vi "scope.vi"() -> ()   [LabVIEW 2017]
uses:
  <vilib>/FPGAPlugInAG/myRIO-1900/niLvFpga_Open_myRIO-1900.vi
  <vilib>/rvi/interface/common/dynamic/niFpgaDynamicAddResources.vi
  <vilib>/rvi/interface/common/niFpgaWaitOnOcc.vi
  <vilib>/Utility/error.llb/Error Cluster From Error Code.vi
  <vilib>/express/express shared/transition.llb/Dynamic To Waveform Array.vi
  <vilib>/express/express signal manip/GetorSetDDTAttributes/Set DDT Attributes/SetT0.vi
  <vilib>/express/express shared/transition.llb/Waveform Array To Dynamic.vi
  <vilib>/rvi/errors/niLvFpgaAdjustHostInterfaceError.vi
  <vilib>/FPGAPlugInAG/Dynamic/niLvFpga_Close_Dynamic.vi
  <vilib>/rvi/interface/nirviOpenFPGA/nirviOpenFPGA.xnode
  FPGA Bitfiles/testznakowarki_FPGATarget_readtescior_VLrWmtzxVOU.lvbitx
  read_and_write.vi
  <vilib>/rvi/interface/nirviMethod/nirviMethod.xnode
  <vilib>/express/express signal manip/GetorSetDDTAttributes/Set DDT Attributes/Set DDT Properties.xnode
  <vilib>/rvi/interface/nirviReadWriteControl/nirviReadWriteControl.xnode
  <vilib>/rvi/interface/nirviCloseFPGA/nirviCloseFPGA.xnode
  <vilib>/rvi/errors/niLvFpgaMergeErrorWithErrorCode.vi
  <vilib>/rvi/interface/Simulation/niFpgaSimulationCallBeginRW.vi
  NiFpgaLv.dll
  <vilib>/FPGAPlugInAG/Dynamic/niLvFpga_ConfigureFifo_Dynamic.vi
  <vilib>/FPGAPlugInAG/Dynamic/niLvFpga_ReadFifo_Dynamic.vi
panel:
  out "Numeric":i32
  out "trigger count queue":i16
  out "inqueue":i32[][](array[numeric])
  in  "stop":bool
  in  "Tab Control":enum32{"now", "data", "settings"}(tab)=enum."settings"
  out "?":string="error now"
  out "error x":bool=TRUE
  out "error y":bool=TRUE
  out "?":string="error now"
  out "max/min x":bool=TRUE
  out "max/min y":bool=TRUE
  out "deviation error x":bool=TRUE
  out "deviation error y":bool=TRUE
  out "data graph":cluster{"time":i32[], "data y":i16[]}[](graph)
  out "template graph":cluster{"time":i32[], "data y":i16[]}[](graph)
  out "size now":i32=2439
  out "max x now":i16=-144
  out "min x now":i16=-150
  out "max y now":i16=116
  out "min y now":i16=-99
  out "template size":i32=10156
  out "template min x":i16=-154
  out "template max x":i16=152
  out "template min y":i16=-135
  out "template max y":i16=139
  out "deviation x":dbl=5341.338663386656
  out "deviation y":dbl=10700.440754407726
  out "template":bool=TRUE
  out "trigger":bool
  out "trigger count":i16=7
  in  "data x":i16[](array[numeric])=[-148, -149, -148, -148, -148, -149, -148, -149, -148, -149, -146, -148, -148, -150, -148, -148, -149, -148, -147, -148, -149, -147, -149, -147, -148, -148, -149, -149, -148, -148, -149, -148, -149, -149, -148, -148, -148, -149, -148, -148, -149, -149, -148, -148, -149, -148, -147, -148, -148, -148, -149, -148, -148, -148, -148, -147, -149, -148, -148, -148, -149, -148, -149, -148, -148, -148, -148, -149, -148, -148, -147, -148, -148, -149, -148, -149, -148, -148, -148, -148, -148, -148, -149, -148, -148, -149, -149, -148, -148, -149, -149, -148, -149, -146, -148, -148, -149, -148, -148, -148, -148, -148, -148, -149, -148, -149, -148, -148, -148, -148, -148, -149, -148, -149, -148, -149, -148, -148, -148, -149, -149, -149, -148, -148, -149, -148, -149, -148, -149, -149, -146, -149, -148, -149, -149, -148, -148, -149, -149, -148, -146, -148, -150, -148, -148, -148, -147, -149, -148, -148, -148, -149, -147, -148, -148, -148, -148, -149, -149, -148, -147, -148, -148, -147, -149, -149, -147, -149, -147, -148, -149, -149, -148, -149, -148, -148, -148, -149, -149, -148, -149, -147, -147, -148, -149, -149, -147, -149, -148, -148, -149, -150, -148, -148, -149, -148, -149, -149, -149, -146, -148, -148, -148, -148, -149, -148, -148, -147, -148, -148, -149, -149, -148, -148, -149, -147, -148, -149, -147, -148, -149, -149, -149, -149, -148, -148, -149, -149, -148, -148, -149, -147, -149, -148, -148, -148, -148, -149, -148, -148, -148, -148, -149, -148, -148, -149, -148, -149, -149, -148, -148, -147, -149, -149, -148, -149, -149, -148, -148, -147, -149, -148, -148, -149, -148, -149, -148, -148, -148, -149, -149, -149, -144, -149, -148, -149, -149, -148, -148, -148, -148, -149, -147, -149, -148, -149, -148, -146, -149, -148, -148, -148, -148, -149, -149, -148, -149, -148, -149, -148, -148, -148, -148, -149, -149, -148, -149, -148, -149, -147, -148, -148, -148, -149, -149, -147, -148, -148, -149, -147, -148, -148, -149, -148, -148, -147, -148, -148, -149, -147, -148, -149, -149, -149, -145, -149, -149, -148, -148, -148, -149, -148, -147, -149, -148, -149, -148, -148, -149, -146, -148, -149, -148, -149, -148, -149, -148, -148, -149, -149, -148, -149, -149, -149, -148, -148, -149, -148, -149, -147, -148, -148, -148, -145, -149, -148, -148, -148, -149, -148, -149, -149, -148, -147, -149, -149, -147, -149, -149, -147, -148, -149, -149, -148, -148, -149, -146, -148, -148, -148, -149, -148, -148, -148, -149, -148, -149, -149, -148, -148, -147, -149, -148, -148, -148, -148, -148, -148, -148, -149, -146, -149, -147, -149, -149, -149, -148, -148, -149, -148, -149, -148, -148, -148, -147, -149, -148, -148, -149, -149, -149, -147, -148, -148, -149, -146, -148, -149, -147, -148, -149, -146, -148, -148, -148, -148, -148, -149, -148, -148, -148, -147, -148, -149, -148, -147, -148, -148, -149, -148, -149, -149, -148, -148, -148, -148, -148, -148, -148, -149, -149, -148, -149, -148, -147, -148, -149, -148, -149, -149, -149, -148, -149, -148, -148, -148, -148, -148, -145, -149, -149, -148, -148, -148, -148, -149, -149, -148, -147, -149, -149, -148, -148, -149, -148, -149, -148, -149, -149, -148, -149, -148, -148, -150, -146, -149, -148, -149, -149, -149, -149, -146, -148, -149, -148, -149, -149, -148, -148, -149, -148, -149, -148, -148, -149, -149, -147, -148, -148, -148, -148, -148, -149, -148, -148, -148, -149, -148, -150, -148, -148, -148, -147, -148, -149, -148, -148, -148, -148, -149, -148, -149, -148, -148, -149, -149, -148, -148, -148, -149, -148, -149, -149, -148, -149, -149, -148, -148, -147, -150, -148, -149, -148, -148, -148, -149, -148, -148, -148, -146, -148, -149, -148, -148, -148, -149, -148, -148, -148, -147, -148, -149, -148, -148, -148, -148, -148, -149, -147, -148, -148, -149, -149, -148, -148, -148, -147, -149, -148, -149, -148, -148, -149, -148, -149, -148, -149, -149, -149, -148, -147, -148, -148, -148, -149, -148, -148, -149, -148, -149, -148, -149, -148, -148, -148, -148, -147, -148, -148, -149, -148, -150, -148, -148, -149, -149, -146, -149, -149, -148, -149, -148, -148, -148, -147, -148, -148, -148, -148, -148, -148, -149, -148, -149, -148, -148, -149, -147, -148, -149, -148, -148, -148, -149, -149, -148, -149, -148, -149, -148, -146, -148, -148, -148, -149, -147, -149, -150, -148, -149, -149, -148, -149, -148, -149, -149, -148, -149, -148, -149, -149, -146, -149, -148, -148, -148, -149, -149, -147, -149, -149, -148, -149, -149, -148, -149, -149, -150, -148, -148, -149, -148, -148, -149, -148, -149, -149, -149, -149, -147, -148, -147, -148, -148, -148, -149, -148, -149, -148, -149, -148, -148, -149, -148, -148, -149, -148, -150, -148, -149, -148, -149, -148, -148, -149, -148, -148, -149, -146, -148, -148, -148, -148, -149, -149, -149, -149, -149, -147, -148, -149, -149, -149, -148, -149, -148, -149, -149, -149, -148, -148, -149, -149, -148, -149, -148, -148, -149, -149, -148, -147, -148, -149, -147, -149, -148, -148, -149, -147, -148, -149, -148, -148, -148, -149, -148, -148, -148, -149, -147, -149, -148, -149, -148, -148, -146, -148, -149, -148, -148, -148, -149, -148, -148, -149, -149, -147, -149, -150, -147, -148, -149, -148, -149, -149, -149, -146, -149, -148, -148, -148, -149, -149, -147, -148, -149, -147, -149, -148, -148, -150, -149, -148, -149, -148, -149, -149, -149, -147, -149, -148, -149, -147, -149, -149, -149, -148, -148, -148, -147, -148, -148, -147, -149, -149, -148, -148, -149, -148, -148, -149, -147, -149, -146, -148, -148, -148, -150, -148, -149, -149, -147, -149, -148, -148, -148, -150, -148, -148, -149, -149, -148, -149, -148, -148, -147, -149, -148, -148, -148, -149, -149, -148, -149, -148, -147, -148, -148, -148, -148, -149, -148, -149, -149, -148, -148, -149, -148, -147, -150, -147, -149, -148, -149, -148, -149, -149, -149, -149, -149, -148, -149, -148, -150, -148, -149, -148, -146, -149, -149, -148, -149, -149, -149, -149, -148, -150, -148, -148, -148, -148, -148, -149, -148, -149, -149, -148, -149, -148, -148, -148, -147, -149, -148, -149, -148, -148, -149, -149, -148, -148, -148, -148, -148, -148, -148, -148, -148, -149, -148, -149, -148, -148, -148, -147, -148, -149, -149, -148, -147, -149, -149, -148, -148, -146, -148, -148, -149, -149, -148, -149, -148, -148, -149, -148, -149, -147, -149, -146, -148, -148, -148, -147, -149, -149, -147, -149, -149, -148, -148, -148, -149, -147, -148, -148, -148, -148, -148, -149, -148, -148, -148, -149, -149, -149, -149, -149, -148, -148, -148, -149, -148, -149, -149, -148, -148, -148, -149, -148, -148, -148, -148, -149, -149, -148, -147, -148, -148, -148, -149, -147, -148, -148, -147, -147, -148, -148, -149, -147, -149, -145, -148, -148, -149, -148, -149, -148, -148, -148, -149, -148, -148, -148, -149, -148, -147, -148, -148, -149, -148, -149, -148, -148, -148, -149, -146, -148, -148, -149, -148, -148, -149, -149, -147, -149, -148, -149, -149, -148, -148, -148, -149, -148, -148, -149, -149, -148, -149, -148, -149, -148, -149, -149, -147, -148, -149, -147, -149, -149, -148, -148, -147, -147, -148, -149, -147, -147, -149, -149, -148, -149, -149, -148, -148, -148, -149, -148, -149, -147, -148, -146, -149, -148, -148, -148, -149, -148, -149, -148, -148, -149, -148, -148, -149, -148, -148, -149, -148, -148, -148, -149, -148, -148, -147, -148, -148, -150, -149, -148, -148, -149, -148, -149, -148, -148, -148, -146, -148, -147, -148, -149, -148, -150, -148, -149, -147, -150, -148, -148, -149, -149, -148, -149, -148, -149, -146, -148, -148, -148, -148, -149, -149, -146, -148, -149, -148, -149, -148, -147, -149, -149, -148, -148, -148, -148, -148, -148, -148, -148, -148, -149, -149, -148, -146, -148, -149, -148, -148, -148, -149, -149, -147, -149, -148, -147, -149, -148, -148, -148, -148, -148, -150, -145, -148, -148, -148, -148, -149, -149, -148, -147, -148, -148, -148, -148, -148, -149, -148, -148, -148, -149, -148, -149, -148, -147, -149, -148, -148, -149, -148, -148, -149, -149, -148, -148, -147, -149, -148, -149, -148, -148, -148, -149, -148, -148, -148, -148, -147, -149, -148, -148, -148, -149, -148, -148, -148, -148, -148, -148, -148, -148, -147, -148, -148, -149, -149, -148, -149, -149, -148, -149, -147, -148, -149, -147, -149, -148, -148, -149, -148, -149, -149, -148, -149, -147, -148, -148, -149, -149, -147, -147, -148, -147, -149, -148, -147, -150, -149, -146, -148, -148, -149, -148, -149, -148, -148, -148, -148, -148, -149, -149, -149, -148, -148, -148, -145, -148, -149, -149, -148, -149, -149, -148, -149, -149, -147, -148, -149, -147, -149, -148, -148, -148, -149, -149, -148, -150, -145, -149, -148, -147, -148, -149, -149, -147, -148, -149, -148, -148, -148, -149, -147, -148, -148, -148, -147, -148, -149, -148, -147, -149, -148, -146, -148, -148, -148, -149, -149, -148, -148, -149, -147, -147, -149, -148, -147, -149, -148, -149, -148, -149, -148, -149, -149, -149, -148, -148, -148, -148, -148, -150, -147, -149, -148, -149, -148, -148, -149, -148, -146, -148, -148, -149, -146, -148, -148, -149, -149, -148, -149, -148, -148, -148, -148, -148, -149, -148, -148, -149, -148, -148, -149, -149, -149, -148, -148, -148, -148, -148, -149, -148, -148, -148, -149, -148, -148, -149, -149, -148, -148, -148, -148, -148, -148, -148, -148, -149, -148, -149, -149, -147, -148, -148, -147, -149, -148, -148, -147, -149, -149, -148, -148, -149, -146, -148, -148, -147, -148, -148, -149, -148, -149, -149, -146, -148, -148, -149, -149, -149, -145, -148, -148, -149, -148, -148, -149, -148, -148, -148, -149, -148, -148, -149, -149, -148, -149, -148, -148, -148, -148, -149, -148, -148, -148, -146, -149, -148, -148, -149, -147, -148, -148, -148, -149, -148, -149, -149, -148, -149, -149, -146, -148, -149, -149, -148, -150, -148, -147, -149, -148, -149, -148, -149, -149, -147, -148, -149, -148, -148, -148, -149, -146, -149, -149, -149, -148, -148, -148, -149, -149, -148, -147, -149, -148, -148, -148, -148, -148, -148, -149, -149, -148, -148, -148, -146, -149, -147, -149, -148, -149, -148, -149, -149, -148, -148, -149, -147, -149, -148, -149, -149, -149, -148, -148, -148, -148, -148, -149, -146, -149, -149, -149, -148, -149, -148, -149, -148, -149, -149, -147, -149, -150, -149, -148, -149, -147, -147, -148, -149, -148, -148, -150, -147, -148, -149, -148, -149, -148, -149, -148, -148, -148, -148, -148, -148, -149, -148, -149, -148, -149, -149, -147, -148, -148, -149, -148, -149, -149, -148, -147, -149, -148, -146, -148, -148, -149, -148, -149, -148, -149, -148, -149, -145, -148, -148, -149, -148, -149, -149, -148, -148, -148, -147, -148, -148, -148, -149, -148, -149, -147, -149, -148, -148, -149, -148, -148, -148, -147, -149, -148, -149, -148, -148, -149, -148, -148, -148, -148, -148, -148, -149, -149, -149, -147, -149, -150, -149, -148, -148, -147, -149, -148, -150, -148, -149, -148, -148, -147, -148, -148, -148, -149, -148, -149, -149, -149, -147, -148, -149, -148, -148, -149, -149, -147, -147, -149, -148, -148, -148, -149, -146, -148, -148, -149, -148, -148, -148, -149, -148, -147, -148, -148, -148, -149, -148, -148, -149, -148, -148, -150, -148, -148, -149, -147, -148, -149, -149, -147, -149, -148, -148, -149, -149, -149, -148, -149, -149, -148, -148, -149, -149, -147, -149, -148, -149, -149, -149, -147, -148, -149, -149, -147, -149, -147, -148, -148, -149, -147, -149, -148, -150, -148, -149, -148, -148, -149, -148, -149, -148, -149, -148, -148, -149, -148, -147, -148, -148, -148, -148, -149, -148, -148, -147, -149, -148, -149, -148, -148, -149, -148, -149, -148, -149, -148, -148, -149, -148, -149, -149, -148, -148, -146, -148, -149, -149, -148, -148, -149, -149, -148, -147, -148, -149, -148, -149, -149, -148, -147, -149, -149, -148, -147, -148, -148, -148, -147, -148, -147, -148, -148, -148, -148, -148, -147, -149, -149, -145, -149, -149, -148, -148, -148, -149, -148, -149, -149, -148, -149, -148, -148, -148, -149, -148, -149, -147, -149, -148, -149, -147, -147, -149, -149, -148, -148, -148, -149, -148, -148, -149, -149, -147, -149, -148, -148, -148, -149, -147, -148, -148, -148, -148, -149, -150, -145, -149, -149, -148, -148, -150, -148, -148, -149, -149, -148, -149, -148, -149, -148, -150, -149, -148, -148, -149, -148, -149, -148, -149, -147, -149, -148, -148, -149, -148, -148, -149, -148, -148, -148, -148, -147, -149, -148, -149, -148, -149, -148, -148, -148, -148, -148, -148, -149, -149, -148, -149, -148, -146, -148, -150, -149, -149, -148, -149, -149, -148, -149, -149, -148, -150, -147, -148, -149, -149, -148, -148, -149, -149, -148, -149, -146, -147, -149, -148, -148, -147, -149, -149, -147, -149, -148, -149, -149, -148, -147, -149, -148, -148, -148, -149, -149, -148, -148, -148, -147, -148, -148, -149, -148, -149, -148, -147, -148, -149, -148, -149, -149, -147, -149, -149, -148, -149, -149, -149, -148, -148, -148, -147, -149, -149, -149, -148, -147, -148, -148, -148, -149, -147, -149, -147, -148, -149, -148, -148, -149, -148, -149, -146, -149, -148, -148, -149, -148, -148, -148, -148, -148, -148, -146, -148, -148, -148, -149, -148, -149, -148, -148, -148, -148, -148, -148, -148, -149, -148, -149, -148, -148, -148, -149, -150, -147, -149, -149, -148, -148, -150, -145, -148, -149, -149, -148, -149, -149, -148, -147, -149, -148, -148, -149, -148, -148, -148, -148, -148, -148, -148, -149, -148, -149, -148, -148, -148, -148, -149, -147, -148, -148, -148, -147, -149, -148, -148, -148, -149, -148, -148, -149, -148, -148, -149, -148, -148, -149, -148, -148, -148, -149, -148, -148, -148, -147, -149, -149, -148, -148, -149, -146, -148, -149, -147, -149, -148, -149, -148, -148, -149, -149, -148, -148, -147, -148, -148, -149, -148, -148, -148, -149, -149, -148, -147, -148, -150, -148, -148, -147, -149, -148, -149, -148, -149, -148, -149, -149, -148, -149, -149, -147, -148, -148, -148, -148, -149, -148, -148, -148, -149, -147, -148, -149, -149, -149, -148, -148, -148, -148, -148, -146, -148, -149, -148, -149, -147, -148, -148, -148, -149, -147, -149, -148, -148, -149, -147, -148, -148, -148, -149, -148, -148, -149, -146, -149, -149, -148, -148, -148, -150, -146, -149, -149, -148, -148, -148, -148, -148, -149, -148, -150, -146, -149, -148, -149, -148, -148, -148, -149, -147, -149, -148, -149, -148, -146, -148, -149, -148, -149, -149, -148, -148, -149, -148, -149, -148, -149, -149, -149, -148, -145, -149, -149, -149, -149, -149, -149, -147, -148, -148, -148, -149, -149, -149, -149, -148, -148, -148, -148, -148, -149, -148, -149, -148, -149, -148, -148, -148, -149, -148, -148, -147, -148, -148, -148, -148, -148, -150, -149, -148, -149, -148, -148, -149, -148, -148, -148, -148, -148, -148, -148, -149, -148, -148, -149, -147, -148, -149, -149, -148, -149, -149, -146, -148, -148, -149, -148, -148, -149, -148, -148, -149, -145, -150]
  in  "data y":i16[](array[numeric])=[-99, -98, -98, -98, -98, -98, -97, -98, -97, -97, -97, -97, -96, -98, -97, -97, -96, -97, -96, -97, -97, -96, -95, -97, -96, -95, -96, -97, -96, -96, -96, -95, -95, -95, -95, -93, -95, -96, -95, -95, -96, -95, -94, -95, -95, -94, -94, -94, -94, -94, -94, -94, -94, -93, -93, -91, -94, -93, -92, -94, -94, -93, -93, -91, -93, -92, -93, -91, -92, -92, -92, -92, -92, -92, -92, -91, -91, -91, -91, -91, -93, -91, -91, -91, -91, -92, -91, -90, -91, -88, -91, -91, -90, -90, -89, -91, -89, -89, -89, -90, -89, -89, -90, -88, -89, -88, -89, -88, -89, -89, -86, -89, -89, -88, -89, -89, -87, -88, -88, -87, -87, -88, -89, -87, -87, -87, -85, -87, -87, -88, -87, -87, -87, -86, -86, -87, -84, -87, -87, -86, -86, -87, -86, -85, -85, -87, -85, -85, -85, -85, -85, -85, -84, -85, -85, -85, -85, -83, -85, -84, -83, -84, -84, -85, -84, -84, -83, -82, -84, -83, -83, -83, -81, -84, -83, -82, -82, -83, -83, -83, -83, -83, -82, -82, -82, -82, -83, -82, -82, -81, -82, -82, -81, -82, -81, -81, -81, -81, -81, -81, -81, -82, -81, -82, -81, -79, -80, -80, -80, -80, -80, -80, -79, -80, -77, -79, -80, -80, -79, -80, -79, -79, -79, -80, -78, -78, -79, -77, -78, -77, -79, -78, -79, -80, -77, -77, -78, -77, -77, -78, -77, -76, -78, -78, -78, -74, -78, -76, -76, -77, -77, -76, -75, -76, -76, -76, -76, -76, -76, -75, -76, -76, -76, -76, -76, -75, -75, -74, -75, -74, -75, -76, -75, -75, -73, -75, -74, -74, -74, -74, -73, -74, -74, -74, -74, -73, -74, -73, -73, -73, -72, -74, -70, -74, -72, -72, -73, -73, -73, -71, -71, -72, -72, -72, -72, -71, -72, -71, -71, -72, -71, -71, -71, -71, -71, -70, -71, -71, -71, -70, -71, -70, -71, -70, -70, -70, -70, -69, -70, -69, -69, -70, -69, -69, -69, -69, -69, -69, -69, -69, -69, -69, -69, -68, -68, -69, -68, -68, -68, -68, -67, -68, -68, -68, -67, -68, -66, -67, -67, -67, -66, -67, -65, -66, -67, -67, -66, -66, -67, -66, -65, -66, -64, -65, -66, -66, -66, -66, -66, -65, -65, -64, -65, -64, -65, -64, -64, -65, -65, -64, -64, -64, -64, -64, -64, -64, -63, -64, -63, -64, -64, -64, -62, -64, -63, -63, -63, -64, -62, -63, -62, -63, -62, -63, -62, -62, -60, -62, -62, -62, -62, -62, -60, -62, -62, -61, -62, -58, -60, -61, -61, -61, -61, -62, -59, -59, -61, -60, -61, -60, -60, -60, -57, -59, -60, -59, -60, -59, -60, -59, -59, -58, -59, -59, -59, -57, -59, -59, -58, -57, -58, -58, -58, -56, -58, -57, -58, -57, -58, -57, -58, -56, -57, -57, -56, -56, -57, -57, -57, -57, -57, -56, -55, -56, -56, -56, -57, -56, -57, -53, -56, -55, -56, -55, -53, -55, -55, -55, -54, -54, -55, -54, -54, -55, -54, -54, -54, -54, -53, -54, -54, -54, -53, -54, -53, -54, -53, -54, -53, -53, -53, -53, -52, -53, -52, -53, -53, -52, -52, -53, -52, -52, -52, -52, -51, -53, -52, -52, -52, -52, -50, -51, -51, -52, -52, -51, -51, -50, -50, -51, -50, -49, -50, -49, -50, -49, -49, -50, -50, -50, -50, -48, -49, -48, -49, -49, -49, -49, -48, -49, -47, -49, -49, -47, -48, -48, -47, -48, -48, -48, -48, -48, -48, -47, -47, -48, -47, -47, -47, -47, -46, -48, -47, -47, -46, -47, -46, -47, -47, -47, -45, -47, -45, -46, -45, -45, -45, -44, -45, -43, -44, -45, -44, -43, -45, -45, -44, -43, -44, -44, -44, -45, -45, -45, -42, -44, -44, -44, -44, -43, -44, -44, -42, -42, -44, -43, -43, -43, -43, -42, -43, -42, -42, -42, -42, -43, -42, -42, -42, -41, -42, -41, -38, -41, -41, -40, -41, -41, -41, -40, -41, -41, -40, -41, -38, -40, -40, -40, -41, -40, -41, -38, -39, -40, -39, -39, -40, -40, -39, -38, -39, -40, -38, -38, -39, -38, -38, -39, -38, -37, -38, -39, -38, -38, -38, -37, -37, -38, -36, -38, -37, -38, -36, -38, -37, -37, -36, -37, -36, -37, -37, -36, -36, -36, -35, -36, -37, -36, -36, -35, -35, -36, -36, -35, -35, -35, -36, -35, -35, -34, -33, -34, -35, -35, -34, -34, -34, -33, -34, -34, -32, -34, -34, -33, -33, -33, -34, -33, -33, -33, -33, -33, -33, -31, -33, -33, -32, -32, -32, -30, -32, -31, -32, -32, -31, -32, -32, -32, -31, -31, -31, -31, -31, -30, -31, -31, -31, -30, -30, -31, -31, -30, -29, -30, -30, -30, -29, -29, -29, -30, -27, -29, -29, -29, -29, -29, -28, -28, -29, -28, -26, -29, -29, -29, -28, -30, -26, -28, -27, -27, -27, -27, -28, -28, -26, -27, -28, -27, -27, -26, -28, -24, -26, -27, -26, -27, -26, -26, -26, -25, -26, -25, -26, -26, -26, -25, -25, -25, -25, -24, -26, -23, -25, -25, -25, -24, -24, -24, -25, -23, -25, -25, -24, -24, -24, -24, -23, -23, -24, -23, -23, -21, -23, -24, -22, -23, -22, -23, -20, -22, -22, -24, -21, -22, -23, -22, -22, -22, -19, -22, -21, -22, -21, -21, -22, -20, -21, -22, -20, -21, -20, -19, -19, -21, -21, -20, -20, -21, -20, -20, -20, -19, -20, -20, -19, -20, -19, -20, -18, -19, -20, -18, -18, -19, -19, -18, -19, -19, -18, -16, -19, -18, -18, -18, -18, -17, -17, -17, -18, -18, -17, -17, -14, -18, -17, -16, -16, -16, -17, -16, -16, -17, -14, -17, -15, -16, -16, -15, -16, -14, -15, -15, -16, -16, -15, -16, -15, -15, -14, -15, -14, -15, -15, -14, -14, -15, -14, -14, -13, -15, -13, -14, -13, -14, -13, -14, -13, -13, -13, -11, -12, -13, -13, -12, -13, -13, -12, -13, -12, -10, -11, -12, -12, -10, -12, -13, -8, -11, -11, -11, -11, -11, -12, -9, -10, -11, -10, -10, -11, -11, -8, -10, -9, -10, -10, -10, -11, -9, -9, -9, -8, -9, -9, -10, -9, -9, -9, -9, -9, -9, -9, -8, -9, -8, -9, -8, -8, -7, -8, -8, -6, -8, -9, -7, -8, -6, -7, -7, -6, -8, -6, -6, -7, -6, -7, -6, -7, -4, -5, -6, -7, -5, -6, -6, -6, -4, -6, -4, -5, -5, -4, -4, -6, -4, -5, -4, -5, -4, -5, -4, -1, -4, -5, -4, -3, -5, -3, -3, -3, -4, -3, -3, -3, -3, -2, -4, -1, -3, -2, -2, -2, -2, -2, -2, -2, -3, -2, -2, -2, -2, -1, 0, -2, -1, -2, -1, -1, -1, -1, -1, -1, 1, 0, -1, -1, 0, -1, -1, -1, 0, -1, 2, 0, 2, 0, 0, 1, 0, 2, 1, 1, 0, 1, 2, 1, 2, 3, 1, 2, 2, 1, 2, 2, 3, 2, 2, 3, 2, 5, 3, 2, 3, 3, 3, 3, 3, 4, 3, 4, 4, 3, 3, 4, 4, 4, 4, 4, 3, 7, 5, 4, 4, 5, 4, 4, 6, 6, 5, 6, 5, 5, 5, 6, 8, 6, 5, 6, 6, 6, 8, 6, 7, 7, 6, 7, 7, 6, 6, 7, 7, 7, 7, 8, 7, 8, 8, 7, 7, 8, 8, 7, 8, 8, 10, 8, 9, 8, 9, 9, 9, 8, 9, 9, 9, 9, 10, 8, 10, 9, 9, 10, 10, 10, 10, 10, 10, 12, 11, 11, 11, 10, 11, 10, 10, 11, 10, 11, 12, 11, 13, 11, 12, 11, 12, 12, 11, 12, 12, 12, 13, 12, 13, 13, 12, 12, 12, 13, 13, 13, 13, 16, 13, 13, 13, 14, 13, 14, 14, 15, 14, 15, 15, 15, 14, 15, 15, 14, 15, 15, 15, 17, 15, 15, 16, 15, 16, 17, 16, 15, 15, 16, 17, 15, 17, 15, 16, 20, 17, 17, 16, 17, 17, 17, 17, 17, 16, 17, 17, 20, 18, 17, 17, 17, 18, 17, 20, 19, 19, 17, 20, 18, 18, 18, 20, 19, 19, 19, 20, 19, 20, 19, 19, 20, 20, 19, 20, 19, 19, 20, 20, 20, 20, 20, 20, 20, 21, 20, 21, 21, 21, 22, 20, 22, 21, 20, 24, 21, 22, 23, 21, 22, 21, 23, 22, 22, 22, 23, 21, 23, 23, 23, 22, 24, 23, 26, 23, 25, 22, 23, 24, 23, 23, 23, 23, 24, 24, 25, 24, 25, 25, 25, 24, 25, 24, 25, 25, 25, 26, 25, 26, 26, 26, 26, 26, 26, 26, 26, 26, 25, 26, 26, 26, 26, 26, 26, 27, 26, 26, 29, 27, 27, 27, 28, 27, 27, 29, 27, 27, 28, 29, 28, 29, 28, 28, 30, 29, 28, 29, 29, 29, 28, 30, 29, 28, 29, 30, 29, 29, 30, 30, 29, 30, 30, 30, 30, 31, 30, 31, 31, 31, 30, 31, 30, 31, 31, 33, 31, 31, 31, 31, 32, 32, 32, 32, 32, 34, 32, 32, 31, 32, 33, 32, 33, 32, 34, 35, 33, 33, 33, 33, 36, 33, 34, 33, 34, 33, 32, 37, 34, 33, 35, 34, 35, 34, 35, 35, 33, 35, 35, 35, 35, 35, 35, 36, 35, 34, 35, 36, 35, 35, 35, 37, 36, 37, 36, 36, 38, 37, 37, 37, 37, 37, 37, 38, 37, 37, 36, 41, 37, 37, 38, 38, 37, 37, 40, 39, 38, 39, 38, 38, 38, 38, 41, 39, 38, 38, 39, 39, 39, 40, 40, 39, 39, 41, 41, 40, 41, 40, 39, 40, 41, 40, 40, 41, 42, 40, 43, 40, 41, 40, 42, 41, 41, 41, 42, 41, 41, 42, 42, 42, 42, 41, 42, 42, 42, 42, 42, 43, 42, 43, 43, 43, 43, 43, 44, 43, 44, 45, 43, 44, 44, 44, 44, 47, 44, 45, 44, 44, 44, 44, 44, 45, 44, 48, 45, 45, 45, 45, 45, 45, 45, 46, 45, 46, 45, 45, 47, 45, 46, 46, 46, 46, 47, 47, 48, 46, 47, 46, 47, 47, 48, 47, 48, 47, 50, 48, 48, 48, 47, 48, 48, 47, 48, 48, 49, 49, 49, 49, 48, 50, 48, 49, 49, 49, 49, 50, 49, 50, 49, 50, 51, 51, 50, 50, 50, 51, 49, 52, 50, 51, 50, 51, 51, 50, 53, 51, 51, 51, 52, 52, 52, 52, 51, 53, 51, 52, 52, 52, 52, 52, 52, 53, 53, 52, 54, 53, 53, 52, 53, 53, 53, 54, 54, 54, 54, 54, 53, 54, 54, 55, 54, 54, 55, 54, 57, 55, 54, 56, 54, 55, 55, 56, 55, 56, 55, 55, 55, 56, 56, 56, 55, 55, 57, 56, 57, 59, 57, 57, 57, 57, 57, 55, 56, 57, 56, 60, 57, 58, 58, 57, 57, 58, 58, 59, 58, 58, 57, 59, 58, 58, 58, 59, 59, 58, 59, 59, 59, 59, 59, 58, 60, 60, 59, 59, 60, 59, 60, 60, 60, 60, 61, 61, 63, 60, 61, 59, 61, 61, 61, 60, 62, 61, 64, 61, 62, 62, 61, 63, 62, 62, 63, 62, 65, 61, 63, 62, 62, 63, 63, 62, 63, 63, 63, 63, 63, 63, 63, 64, 63, 64, 64, 64, 63, 66, 64, 64, 64, 64, 64, 64, 65, 66, 64, 68, 65, 65, 66, 66, 65, 65, 66, 65, 64, 67, 66, 65, 66, 66, 65, 67, 67, 66, 67, 66, 67, 66, 67, 69, 67, 67, 68, 68, 68, 68, 68, 67, 68, 67, 68, 67, 68, 68, 68, 68, 69, 68, 69, 70, 69, 69, 70, 69, 68, 71, 69, 69, 70, 69, 69, 69, 71, 70, 70, 71, 70, 69, 70, 72, 71, 70, 71, 72, 71, 71, 73, 71, 72, 72, 71, 73, 71, 74, 72, 72, 73, 72, 72, 72, 72, 73, 71, 73, 72, 72, 74, 73, 73, 73, 73, 74, 74, 73, 74, 73, 75, 73, 74, 74, 73, 74, 75, 73, 75, 74, 75, 74, 75, 74, 75, 75, 76, 75, 75, 76, 75, 75, 76, 78, 75, 76, 77, 76, 76, 76, 76, 76, 76, 77, 76, 76, 77, 78, 77, 77, 77, 77, 77, 78, 77, 77, 77, 78, 78, 79, 79, 78, 79, 78, 79, 78, 79, 81, 78, 79, 78, 79, 79, 80, 79, 81, 78, 80, 80, 80, 79, 80, 80, 81, 80, 80, 81, 80, 81, 81, 80, 80, 82, 81, 81, 81, 82, 80, 82, 81, 82, 84, 83, 81, 82, 82, 82, 82, 84, 82, 82, 82, 83, 82, 82, 85, 83, 83, 83, 84, 83, 83, 86, 83, 84, 84, 83, 84, 83, 85, 84, 84, 84, 84, 84, 85, 85, 85, 86, 87, 85, 85, 85, 85, 85, 86, 85, 86, 88, 86, 85, 86, 86, 85, 86, 86, 87, 87, 87, 87, 86, 86, 87, 87, 87, 88, 87, 88, 87, 90, 87, 88, 88, 87, 88, 88, 88, 88, 90, 91, 89, 88, 89, 90, 88, 89, 89, 90, 90, 89, 90, 90, 89, 90, 89, 91, 89, 90, 90, 90, 90, 90, 91, 90, 91, 91, 92, 90, 91, 91, 90, 91, 92, 91, 92, 92, 91, 92, 92, 93, 91, 92, 92, 92, 92, 92, 95, 93, 93, 93, 92, 93, 93, 93, 93, 93, 94, 93, 93, 96, 94, 94, 94, 94, 94, 94, 94, 95, 94, 95, 95, 94, 94, 95, 94, 96, 94, 99, 95, 96, 96, 95, 96, 97, 96, 98, 96, 95, 96, 97, 96, 96, 97, 96, 96, 97, 96, 96, 98, 97, 98, 97, 98, 98, 98, 98, 97, 97, 99, 97, 99, 98, 98, 98, 99, 99, 98, 101, 99, 98, 98, 99, 99, 99, 101, 99, 100, 99, 99, 100, 99, 101, 100, 100, 100, 101, 101, 102, 101, 102, 100, 101, 100, 100, 101, 101, 101, 104, 101, 101, 102, 102, 102, 102, 102, 101, 101, 104, 103, 102, 102, 103, 102, 103, 103, 103, 102, 104, 103, 104, 102, 103, 103, 102, 104, 104, 104, 104, 103, 104, 104, 104, 104, 104, 104, 104, 104, 105, 106, 105, 105, 105, 105, 105, 107, 105, 105, 105, 106, 105, 106, 106, 106, 106, 110, 106, 106, 105, 108, 106, 108, 107, 107, 108, 107, 107, 107, 107, 108, 107, 108, 109, 107, 108, 109, 108, 108, 109, 108, 110, 108, 110, 109, 110, 108, 110, 109, 109, 108, 110, 109, 110, 109, 110, 109, 109, 110, 110, 111, 110, 110, 110, 110, 111, 111, 111, 110, 111, 111, 113, 111, 111, 111, 112, 111, 111, 112, 112, 112, 113, 112, 112, 112, 111, 116, 112, 113, 113, 112, 113, 113, 112, 113, 113, 114, 113, 115, 114, 114, 113, 115, 114, 113, 114, 114]
  in  "template x":i16[](array[numeric])=array[10156 elements]
  in  "template y":i16[](array[numeric])=array[10156 elements]
  in  "time":i32[](array[numeric])=[0, 1, 2, 3, 4, 5, 6, 7, 8, 9, 10, 11, 12, 13, 14, 15, 16, 17, 18, 19, 20, 21, 22, 23, 24, 25, 26, 27, 28, 29, 30, 31, 32, 33, 34, 35, 36, 37, 38, 39, 40, 41, 42, 43, 44, 45, 46, 47, 48, 49, 50, 51, 52, 53, 54, 55, 56, 57, 58, 59, 60, 61, 62, 63, 64, 65, 66, 67, 68, 69, 70, 71, 72, 73, 74, 75, 76, 77, 78, 79, 80, 81, 82, 83, 84, 85, 86, 87, 88, 89, 90, 91, 92, 93, 94, 95, 96, 97, 98, 99, 100, 101, 102, 103, 104, 105, 106, 107, 108, 109, 110, 111, 112, 113, 114, 115, 116, 117, 118, 119, 120, 121, 122, 123, 124, 125, 126, 127, 128, 129, 130, 131, 132, 133, 134, 135, 136, 137, 138, 139, 140, 141, 142, 143, 144, 145, 146, 147, 148, 149, 150, 151, 152, 153, 154, 155, 156, 157, 158, 159, 160, 161, 162, 163, 164, 165, 166, 167, 168, 169, 170, 171, 172, 173, 174, 175, 176, 177, 178, 179, 180, 181, 182, 183, 184, 185, 186, 187, 188, 189, 190, 191, 192, 193, 194, 195, 196, 197, 198, 199, 200, 201, 202, 203, 204, 205, 206, 207, 208, 209, 210, 211, 212, 213, 214, 215, 216, 217, 218, 219, 220, 221, 222, 223, 224, 225, 226, 227, 228, 229, 230, 231, 232, 233, 234, 235, 236, 237, 238, 239, 240, 241, 242, 243, 244, 245, 246, 247, 248, 249, 250, 251, 252, 253, 254, 255, 256, 257, 258, 259, 260, 261, 262, 263, 264, 265, 266, 267, 268, 269, 270, 271, 272, 273, 274, 275, 276, 277, 278, 279, 280, 281, 282, 283, 284, 285, 286, 287, 288, 289, 290, 291, 292, 293, 294, 295, 296, 297, 298, 299, 300, 301, 302, 303, 304, 305, 306, 307, 308, 309, 310, 311, 312, 313, 314, 315, 316, 317, 318, 319, 320, 321, 322, 323, 324, 325, 326, 327, 328, 329, 330, 331, 332, 333, 334, 335, 336, 337, 338, 339, 340, 341, 342, 343, 344, 345, 346, 347, 348, 349, 350, 351, 352, 353, 354, 355, 356, 357, 358, 359, 360, 361, 362, 363, 364, 365, 366, 367, 368, 369, 370, 371, 372, 373, 374, 375, 376, 377, 378, 379, 380, 381, 382, 383, 384, 385, 386, 387, 388, 389, 390, 391, 392, 393, 394, 395, 396, 397, 398, 399, 400, 401, 402, 403, 404, 405, 406, 407, 408, 409, 410, 411, 412, 413, 414, 415, 416, 417, 418, 419, 420, 421, 422, 423, 424, 425, 426, 427, 428, 429, 430, 431, 432, 433, 434, 435, 436, 437, 438, 439, 440, 441, 442, 443, 444, 445, 446, 447, 448, 449, 450, 451, 452, 453, 454, 455, 456, 457, 458, 459, 460, 461, 462, 463, 464, 465, 466, 467, 468, 469, 470, 471, 472, 473, 474, 475, 476, 477, 478, 479, 480, 481, 482, 483, 484, 485, 486, 487, 488, 489, 490, 491, 492, 493, 494, 495, 496, 497, 498, 499, 500, 501, 502, 503, 504, 505, 506, 507, 508, 509, 510, 511, 512, 513, 514, 515, 516, 517, 518, 519, 520, 521, 522, 523, 524, 525, 526, 527, 528, 529, 530, 531, 532, 533, 534, 535, 536, 537, 538, 539, 540, 541, 542, 543, 544, 545, 546, 547, 548, 549, 550, 551, 552, 553, 554, 555, 556, 557, 558, 559, 560, 561, 562, 563, 564, 565, 566, 567, 568, 569, 570, 571, 572, 573, 574, 575, 576, 577, 578, 579, 580, 581, 582, 583, 584, 585, 586, 587, 588, 589, 590, 591, 592, 593, 594, 595, 596, 597, 598, 599, 600, 601, 602, 603, 604, 605, 606, 607, 608, 609, 610, 611, 612, 613, 614, 615, 616, 617, 618, 619, 620, 621, 622, 623, 624, 625, 626, 627, 628, 629, 630, 631, 632, 633, 634, 635, 636, 637, 638, 639, 640, 641, 642, 643, 644, 645, 646, 647, 648, 649, 650, 651, 652, 653, 654, 655, 656, 657, 658, 659, 660, 661, 662, 663, 664, 665, 666, 667, 668, 669, 670, 671, 672, 673, 674, 675, 676, 677, 678, 679, 680, 681, 682, 683, 684, 685, 686, 687, 688, 689, 690, 691, 692, 693, 694, 695, 696, 697, 698, 699, 700, 701, 702, 703, 704, 705, 706, 707, 708, 709, 710, 711, 712, 713, 714, 715, 716, 717, 718, 719, 720, 721, 722, 723, 724, 725, 726, 727, 728, 729, 730, 731, 732, 733, 734, 735, 736, 737, 738, 739, 740, 741, 742, 743, 744, 745, 746, 747, 748, 749, 750, 751, 752, 753, 754, 755, 756, 757, 758, 759, 760, 761, 762, 763, 764, 765, 766, 767, 768, 769, 770, 771, 772, 773, 774, 775, 776, 777, 778, 779, 780, 781, 782, 783, 784, 785, 786, 787, 788, 789, 790, 791, 792, 793, 794, 795, 796, 797, 798, 799, 800, 801, 802, 803, 804, 805, 806, 807, 808, 809, 810, 811, 812, 813, 814, 815, 816, 817, 818, 819, 820, 821, 822, 823, 824, 825, 826, 827, 828, 829, 830, 831, 832, 833, 834, 835, 836, 837, 838, 839, 840, 841, 842, 843, 844, 845, 846, 847, 848, 849, 850, 851, 852, 853, 854, 855, 856, 857, 858, 859, 860, 861, 862, 863, 864, 865, 866, 867, 868, 869, 870, 871, 872, 873, 874, 875, 876, 877, 878, 879, 880, 881, 882, 883, 884, 885, 886, 887, 888, 889, 890, 891, 892, 893, 894, 895, 896, 897, 898, 899, 900, 901, 902, 903, 904, 905, 906, 907, 908, 909, 910, 911, 912, 913, 914, 915, 916, 917, 918, 919, 920, 921, 922, 923, 924, 925, 926, 927, 928, 929, 930, 931, 932, 933, 934, 935, 936, 937, 938, 939, 940, 941, 942, 943, 944, 945, 946, 947, 948, 949, 950, 951, 952, 953, 954, 955, 956, 957, 958, 959, 960, 961, 962, 963, 964, 965, 966, 967, 968, 969, 970, 971, 972, 973, 974, 975, 976, 977, 978, 979, 980, 981, 982, 983, 984, 985, 986, 987, 988, 989, 990, 991, 992, 993, 994, 995, 996, 997, 998, 999, 1000, 1001, 1002, 1003, 1004, 1005, 1006, 1007, 1008, 1009, 1010, 1011, 1012, 1013, 1014, 1015, 1016, 1017, 1018, 1019, 1020, 1021, 1022, 1023, 1024, 1025, 1026, 1027, 1028, 1029, 1030, 1031, 1032, 1033, 1034, 1035, 1036, 1037, 1038, 1039, 1040, 1041, 1042, 1043, 1044, 1045, 1046, 1047, 1048, 1049, 1050, 1051, 1052, 1053, 1054, 1055, 1056, 1057, 1058, 1059, 1060, 1061, 1062, 1063, 1064, 1065, 1066, 1067, 1068, 1069, 1070, 1071, 1072, 1073, 1074, 1075, 1076, 1077, 1078, 1079, 1080, 1081, 1082, 1083, 1084, 1085, 1086, 1087, 1088, 1089, 1090, 1091, 1092, 1093, 1094, 1095, 1096, 1097, 1098, 1099, 1100, 1101, 1102, 1103, 1104, 1105, 1106, 1107, 1108, 1109, 1110, 1111, 1112, 1113, 1114, 1115, 1116, 1117, 1118, 1119, 1120, 1121, 1122, 1123, 1124, 1125, 1126, 1127, 1128, 1129, 1130, 1131, 1132, 1133, 1134, 1135, 1136, 1137, 1138, 1139, 1140, 1141, 1142, 1143, 1144, 1145, 1146, 1147, 1148, 1149, 1150, 1151, 1152, 1153, 1154, 1155, 1156, 1157, 1158, 1159, 1160, 1161, 1162, 1163, 1164, 1165, 1166, 1167, 1168, 1169, 1170, 1171, 1172, 1173, 1174, 1175, 1176, 1177, 1178, 1179, 1180, 1181, 1182, 1183, 1184, 1185, 1186, 1187, 1188, 1189, 1190, 1191, 1192, 1193, 1194, 1195, 1196, 1197, 1198, 1199, 1200, 1201, 1202, 1203, 1204, 1205, 1206, 1207, 1208, 1209, 1210, 1211, 1212, 1213, 1214, 1215, 1216, 1217, 1218, 1219, 1220, 1221, 1222, 1223, 1224, 1225, 1226, 1227, 1228, 1229, 1230, 1231, 1232, 1233, 1234, 1235, 1236, 1237, 1238, 1239, 1240, 1241, 1242, 1243, 1244, 1245, 1246, 1247, 1248, 1249, 1250, 1251, 1252, 1253, 1254, 1255, 1256, 1257, 1258, 1259, 1260, 1261, 1262, 1263, 1264, 1265, 1266, 1267, 1268, 1269, 1270, 1271, 1272, 1273, 1274, 1275, 1276, 1277, 1278, 1279, 1280, 1281, 1282, 1283, 1284, 1285, 1286, 1287, 1288, 1289, 1290, 1291, 1292, 1293, 1294, 1295, 1296, 1297, 1298, 1299, 1300, 1301, 1302, 1303, 1304, 1305, 1306, 1307, 1308, 1309, 1310, 1311, 1312, 1313, 1314, 1315, 1316, 1317, 1318, 1319, 1320, 1321, 1322, 1323, 1324, 1325, 1326, 1327, 1328, 1329, 1330, 1331, 1332, 1333, 1334, 1335, 1336, 1337, 1338, 1339, 1340, 1341, 1342, 1343, 1344, 1345, 1346, 1347, 1348, 1349, 1350, 1351, 1352, 1353, 1354, 1355, 1356, 1357, 1358, 1359, 1360, 1361, 1362, 1363, 1364, 1365, 1366, 1367, 1368, 1369, 1370, 1371, 1372, 1373, 1374, 1375, 1376, 1377, 1378, 1379, 1380, 1381, 1382, 1383, 1384, 1385, 1386, 1387, 1388, 1389, 1390, 1391, 1392, 1393, 1394, 1395, 1396, 1397, 1398, 1399, 1400, 1401, 1402, 1403, 1404, 1405, 1406, 1407, 1408, 1409, 1410, 1411, 1412, 1413, 1414, 1415, 1416, 1417, 1418, 1419, 1420, 1421, 1422, 1423, 1424, 1425, 1426, 1427, 1428, 1429, 1430, 1431, 1432, 1433, 1434, 1435, 1436, 1437, 1438, 1439, 1440, 1441, 1442, 1443, 1444, 1445, 1446, 1447, 1448, 1449, 1450, 1451, 1452, 1453, 1454, 1455, 1456, 1457, 1458, 1459, 1460, 1461, 1462, 1463, 1464, 1465, 1466, 1467, 1468, 1469, 1470, 1471, 1472, 1473, 1474, 1475, 1476, 1477, 1478, 1479, 1480, 1481, 1482, 1483, 1484, 1485, 1486, 1487, 1488, 1489, 1490, 1491, 1492, 1493, 1494, 1495, 1496, 1497, 1498, 1499, 1500, 1501, 1502, 1503, 1504, 1505, 1506, 1507, 1508, 1509, 1510, 1511, 1512, 1513, 1514, 1515, 1516, 1517, 1518, 1519, 1520, 1521, 1522, 1523, 1524, 1525, 1526, 1527, 1528, 1529, 1530, 1531, 1532, 1533, 1534, 1535, 1536, 1537, 1538, 1539, 1540, 1541, 1542, 1543, 1544, 1545, 1546, 1547, 1548, 1549, 1550, 1551, 1552, 1553, 1554, 1555, 1556, 1557, 1558, 1559, 1560, 1561, 1562, 1563, 1564, 1565, 1566, 1567, 1568, 1569, 1570, 1571, 1572, 1573, 1574, 1575, 1576, 1577, 1578, 1579, 1580, 1581, 1582, 1583, 1584, 1585, 1586, 1587, 1588, 1589, 1590, 1591, 1592, 1593, 1594, 1595, 1596, 1597, 1598, 1599, 1600, 1601, 1602, 1603, 1604, 1605, 1606, 1607, 1608, 1609, 1610, 1611, 1612, 1613, 1614, 1615, 1616, 1617, 1618, 1619, 1620, 1621, 1622, 1623, 1624, 1625, 1626, 1627, 1628, 1629, 1630, 1631, 1632, 1633, 1634, 1635, 1636, 1637, 1638, 1639, 1640, 1641, 1642, 1643, 1644, 1645, 1646, 1647, 1648, 1649, 1650, 1651, 1652, 1653, 1654, 1655, 1656, 1657, 1658, 1659, 1660, 1661, 1662, 1663, 1664, 1665, 1666, 1667, 1668, 1669, 1670, 1671, 1672, 1673, 1674, 1675, 1676, 1677, 1678, 1679, 1680, 1681, 1682, 1683, 1684, 1685, 1686, 1687, 1688, 1689, 1690, 1691, 1692, 1693, 1694, 1695, 1696, 1697, 1698, 1699, 1700, 1701, 1702, 1703, 1704, 1705, 1706, 1707, 1708, 1709, 1710, 1711, 1712, 1713, 1714, 1715, 1716, 1717, 1718, 1719, 1720, 1721, 1722, 1723, 1724, 1725, 1726, 1727, 1728, 1729, 1730, 1731, 1732, 1733, 1734, 1735, 1736, 1737, 1738, 1739, 1740, 1741, 1742, 1743, 1744, 1745, 1746, 1747, 1748, 1749, 1750, 1751, 1752, 1753, 1754, 1755, 1756, 1757, 1758, 1759, 1760, 1761, 1762, 1763, 1764, 1765, 1766, 1767, 1768, 1769, 1770, 1771, 1772, 1773, 1774, 1775, 1776, 1777, 1778, 1779, 1780, 1781, 1782, 1783, 1784, 1785, 1786, 1787, 1788, 1789, 1790, 1791, 1792, 1793, 1794, 1795, 1796, 1797, 1798, 1799, 1800, 1801, 1802, 1803, 1804, 1805, 1806, 1807, 1808, 1809, 1810, 1811, 1812, 1813, 1814, 1815, 1816, 1817, 1818, 1819, 1820, 1821, 1822, 1823, 1824, 1825, 1826, 1827, 1828, 1829, 1830, 1831, 1832, 1833, 1834, 1835, 1836, 1837, 1838, 1839, 1840, 1841, 1842, 1843, 1844, 1845, 1846, 1847, 1848, 1849, 1850, 1851, 1852, 1853, 1854, 1855, 1856, 1857, 1858, 1859, 1860, 1861, 1862, 1863, 1864, 1865, 1866, 1867, 1868, 1869, 1870, 1871, 1872, 1873, 1874, 1875, 1876, 1877, 1878, 1879, 1880, 1881, 1882, 1883, 1884, 1885, 1886, 1887, 1888, 1889, 1890, 1891, 1892, 1893, 1894, 1895, 1896, 1897, 1898, 1899, 1900, 1901, 1902, 1903, 1904, 1905, 1906, 1907, 1908, 1909, 1910, 1911, 1912, 1913, 1914, 1915, 1916, 1917, 1918, 1919, 1920, 1921, 1922, 1923, 1924, 1925, 1926, 1927, 1928, 1929, 1930, 1931, 1932, 1933, 1934, 1935, 1936, 1937, 1938, 1939, 1940, 1941, 1942, 1943, 1944, 1945, 1946, 1947, 1948, 1949, 1950, 1951, 1952, 1953, 1954, 1955, 1956, 1957, 1958, 1959, 1960, 1961, 1962, 1963, 1964, 1965, 1966, 1967, 1968, 1969, 1970, 1971, 1972, 1973, 1974, 1975, 1976, 1977, 1978, 1979, 1980, 1981, 1982, 1983, 1984, 1985, 1986, 1987, 1988, 1989, 1990, 1991, 1992, 1993, 1994, 1995, 1996, 1997, 1998, 1999, 2000, 2001, 2002, 2003, 2004, 2005, 2006, 2007, 2008, 2009, 2010, 2011, 2012, 2013, 2014, 2015, 2016, 2017, 2018, 2019, 2020, 2021, 2022, 2023, 2024, 2025, 2026, 2027, 2028, 2029, 2030, 2031, 2032, 2033, 2034, 2035, 2036, 2037, 2038, 2039, 2040, 2041, 2042, 2043, 2044, 2045, 2046, 2047, 2048, 2049, 2050, 2051, 2052, 2053, 2054, 2055, 2056, 2057, 2058, 2059, 2060, 2061, 2062, 2063, 2064, 2065, 2066, 2067, 2068, 2069, 2070, 2071, 2072, 2073, 2074, 2075, 2076, 2077, 2078, 2079, 2080, 2081, 2082, 2083, 2084, 2085, 2086, 2087, 2088, 2089, 2090, 2091, 2092, 2093, 2094, 2095, 2096, 2097, 2098, 2099, 2100, 2101, 2102, 2103, 2104, 2105, 2106, 2107, 2108, 2109, 2110, 2111, 2112, 2113, 2114, 2115, 2116, 2117, 2118, 2119, 2120, 2121, 2122, 2123, 2124, 2125, 2126, 2127, 2128, 2129, 2130, 2131, 2132, 2133, 2134, 2135, 2136, 2137, 2138, 2139, 2140, 2141, 2142, 2143, 2144, 2145, 2146, 2147, 2148, 2149, 2150, 2151, 2152, 2153, 2154, 2155, 2156, 2157, 2158, 2159, 2160, 2161, 2162, 2163, 2164, 2165, 2166, 2167, 2168, 2169, 2170, 2171, 2172, 2173, 2174, 2175, 2176, 2177, 2178, 2179, 2180, 2181, 2182, 2183, 2184, 2185, 2186, 2187, 2188, 2189, 2190, 2191, 2192, 2193, 2194, 2195, 2196, 2197, 2198, 2199, 2200, 2201, 2202, 2203, 2204, 2205, 2206, 2207, 2208, 2209, 2210, 2211, 2212, 2213, 2214, 2215, 2216, 2217, 2218, 2219, 2220, 2221, 2222, 2223, 2224, 2225, 2226, 2227, 2228, 2229, 2230, 2231, 2232, 2233, 2234, 2235, 2236, 2237, 2238, 2239, 2240, 2241, 2242, 2243, 2244, 2245, 2246, 2247, 2248, 2249, 2250, 2251, 2252, 2253, 2254, 2255, 2256, 2257, 2258, 2259, 2260, 2261, 2262, 2263, 2264, 2265, 2266, 2267, 2268, 2269, 2270, 2271, 2272, 2273, 2274, 2275, 2276, 2277, 2278, 2279, 2280, 2281, 2282, 2283, 2284, 2285, 2286, 2287, 2288, 2289, 2290, 2291, 2292, 2293, 2294, 2295, 2296, 2297, 2298, 2299, 2300, 2301, 2302, 2303, 2304, 2305, 2306, 2307, 2308, 2309, 2310, 2311, 2312, 2313, 2314, 2315, 2316, 2317, 2318, 2319, 2320, 2321, 2322, 2323, 2324, 2325, 2326, 2327, 2328, 2329, 2330, 2331, 2332, 2333, 2334, 2335, 2336, 2337, 2338, 2339, 2340, 2341, 2342, 2343, 2344, 2345, 2346, 2347, 2348, 2349, 2350, 2351, 2352, 2353, 2354, 2355, 2356, 2357, 2358, 2359, 2360, 2361, 2362, 2363, 2364, 2365, 2366, 2367, 2368, 2369, 2370, 2371, 2372, 2373, 2374, 2375, 2376, 2377, 2378, 2379, 2380, 2381, 2382, 2383, 2384, 2385, 2386, 2387, 2388, 2389, 2390, 2391, 2392, 2393, 2394, 2395, 2396, 2397, 2398, 2399, 2400, 2401, 2402, 2403, 2404, 2405, 2406, 2407, 2408, 2409, 2410, 2411, 2412, 2413, 2414, 2415, 2416, 2417, 2418, 2419, 2420, 2421, 2422, 2423, 2424, 2425, 2426, 2427, 2428, 2429, 2430, 2431, 2432, 2433, 2434, 2435, 2436, 2437, 2438]
  out "pwm now":u16[](array[numeric])
  out "x now":i16[](array[numeric])=[-1, 0, -2, -1, -1, -1, -1, -1, -1, 0, -2, 0, -1, -1, -1, -1, -2, -1, -1, 1, -2, -1, -1, -2, -1, -1, -2, -1, 0, -1, -1, -1, -1, -1, -1, -2, -2, -1, -2, 0, 0, -1, -2, -1, -1, -1, -1, 0, -1, -1, -1, -1, -1, -1, -1, -2, -2, -1, -1, -1, -1, -1, -1, -2, 1, -1, -1, -2, -1, -1, -1, -1, -1, -1, -1, -2, -1, 0, -2, -1, 0, -2, -1, -1, -1, 0, -1, -1, 0, -2, 0, -1, -1, -1, -1, 0, 0, -1, 0, -1, 0, -1, 0, 0, -1, -1, 0, -1, -2, -1, -1, -1, -1, -1, 0, -2, 0, -2, -1, -1, -2, -2, 0, -1, -1, 1, -1, -1, -2, 0, -1, 0, -1, -1, -2, 0, -1, -1, -1, -1, -1, 0, -1, -1, -2, -1, -1, -1, 0, -1, -1, -2, -1, -1, -1, 0, -1, -2, 0, -1, -1, -1, 0, 0, -1, -1, -1, -1, -1, -1, -1, -2, -1, 0, -1, -1, -1, -1, -1, -1, -2, 2, -1, -1, -1, -1, -1, -1, -1, -1, -1, 0, -1, -1, -1, -1, 0, -2, -1, -1, -1, -1, -1, -1, -1, 0, -1, -1, 0, -2, 0, -2, -1, -1, 0, -1, 0, -2, 0, -1, -1, 1, -1, -1, 0, -1, -1, -1, 0, -1, -2, -1, -1, -2, 0, -1, -1, -1, -1, -1, -1, 0, -1, -1, -1, -1, 1, -1, -1, -1, -1, -1, -1, -2, 0, -1, -1, -1, 0, -1, -1, -1, -1, -2, -1, -1, -1, -1, -1, -1, -1, 0, -1, -1, -1, 0, -1, 1, -1, -1, -2, -1, -1, -1, -1, -1, -1, -1, -1, -1, -1, -1, 0, -2, -1, -1, -1, -1, -2, 1, -1, -2, -1, 0, -2, -1, 1, 0, -1, -1, -1, -1, -1, -1, -1, -1, -1, 0, -1, -1, -1, -1, -1, 0, -1, -1, -1, 0, -1, -1, -1, -1, -2, -1, -1, -1, -1, 2, -1, 0, 0, -1, -2, -1, 1, -1, -1, 0, -2, -1, -1, -1, 0, -1, -1, -1, -1, 0, -1, 0, -1, -1, -1, 0, -2, -1, -2, -1, -1, 0, -1, -1, -1, 1, -1, -2, -1, -1, -1, -1, -1, -1, -1, -1, -1, -1, 0, -2, -1, -1, 0, -1, -1, -1, 0, -2, -1, 1, -1, -1, -1, -1, -1, 0, -1, -1, -1, -1, -1, 0, -1, -1, 0, -1, -1, 0, 0, -1, 0, 0, -2, -1, -1, -1, -1, 0, 1, -1, -1, -1, -1, -1, 0, -1, -2, -1, -1, -1, 0, -1, -1, -1, 0, -1, -1, -1, -1, -2, -1, 0, 0, -1, -1, 0, -1, -1, -1, -1, -1, 0, -1, -1, -1, -2, -1, -1, -1, -1, -1, -1, -1, -1, -2, -2, -1, -1, -1, -1, -1, 0, -2, -1, -1, 0, -1, -1, -2, -1, 0, -1, 0, 0, -1, -2, -2, -1, -2, 0, -1, 1, -1, -1, -2, -1, -1, -1, -1, 0, -2, -1, -1, -1, 0, 0, -1, -1, -1, 0, -2, 0, -1, -1, 0, 0, -1, -1, -1, -1, -1, -1, 0, -1, -2, 0, -1, 0, -1, 0, -1, -1, -1, -1, -1, 0, -1, -2, 0, 0, -2, -1, -1, -1, -2, 0, -1, -2, -1, -1, -1, 0, -1, 0, -1, 0, -1, -1, -1, -1, -2, -1, -1, -1, 1, -1, -1, -1, -1, -1, -1, -1, -1, -1, 0, -1, -1, 0, -1, -1, -1, -1, -1, -1, -1, -1, -1, 1, -1, -1, 0, -1, -1, -1, -1, -1, -3, -1, -2, -1, 1, -1, -1, 0, -1, -1, -2, 0, -2, -1, 1, -1, -1, -1, -1, -1, -1, 0, -1, -1, -1, -1, -1, -1, 1, -1, -1, 0, -2, -1, -1, -2, -1, 0, -1, -1, -1, 0, -1, -1, -1, -1, -1, 0, -1, -1, -2, 0, -1, -1, 0, -1, -1, -1, -1, -1, 0, -1, -1, -1, -1, -2, 0, -1, -2, -1, -1, -1, -2, 0, -1, -1, -1, -1, -1, -1, 0, 0, -2, -1, -1, -1, 0, 0, -1, -3, 1, -1, -1, -1, -1, -2, -1, -1, -1, -2, 1, -1, -1, -1, -1, -1, -1, -1, -1, -1, -1, -1, 0, -1, -1, -1, -1, 0, -2, 1, -1, -1, -1, 0, -1, -2, 1, -1, 0, -2, 0, -1, -1, -1, -1, -1, -1, -1, -1, -1, 0, -1, -1, 0, -1, -1, -1, -1, -1, -1, 0, -1, -1, -1, -1, -2, -1, 0, -1, -1, -2, -1, -1, -2, 0, -1, -1, -1, -1, -1, -2, -1, 0, -1, -1, -1, -2, 0, 0, -1, -1, -1, -1, -1, -1, -1, 0, 0, -1, -1, -1, -1, -1, -1, -1, 0]
  out "y now":i16[](array[numeric])=[-2, -1, -2, -1, -1, 2, -1, -2, -2, -1, -3, -1, -2, -2, -1, -2, -2, -1, -2, -1, -1, -2, -2, -2, -1, -1, -2, -1, 1, -1, -1, -3, -1, -2, -1, -1, -1, -2, -1, -2, -1, 0, -1, -2, -1, -1, -1, -1, -2, -2, -2, 1, -2, -1, -1, -1, -2, -1, -2, -1, -2, -2, -1, -1, -1, -2, -1, -1, -2, -1, -1, -1, -1, -1, -1, -2, -1, -1, 0, -1, 0, -1, -1, -1, -1, -1, -2, -3, -1, -1, -1, 0, -2, -1, -2, -1, -1, -1, -1, -2, -1, 3, -1, -1, -1, -2, -1, -2, 0, -1, -1, -1, -1, -2, -1, -1, -1, -1, -2, -1, -1, -1, -1, -2, 1, -1, -1, -1, -2, -2, -2, -2, -1, -2, -1, -1, -1, 1, -2, -1, -2, -2, -2, -1, -2, 0, -2, 1, 0, -1, -2, -1, -3, 1, -2, -1, -1, -1, -1, -1, -1, 0, -1, -2, -1, -1, -2, -2, -1, -2, -1, -1, -1, -2, -1, -1, -2, 0, -2, -1, -2, -1, -1, -2, -2, -1, -2, -1, -1, -1, -1, -1, -1, -1, -1, -1, -2, -2, -1, -1, -1, -1, -2, -2, -1, -2, 0, -1, -1, -2, -2, -1, -3, 0, -1, -2, -1, -2, -1, -2, -1, -1, -2, -1, -1, -2, -1, -1, -1, -1, -1, -1, -1, 0, -1, -1, -2, -1, -2, -2, -1, -1, -2, -2, 0, -2, -2, -1, -1, -2, -2, -1, -2, -2, -1, -2, -1, -2, -1, -1, -1, -1, -1, -1, 0, -2, -1, -2, -1, -2, -1, -1, -2, 0, -1, -2, -1, -1, -1, -3, -1, -1, -2, 0, 0, -2, -1, -1, -1, -2, -2, -1, -2, -1, -1, -2, -1, -1, -2, -2, -1, -1, -2, -2, 0, -1, -2, -1, -1, -2, -2, -1, -2, -1, -1, -2, -2, -1, -1, 0, -1, -1, -2, -1, -1, -1, -1, -1, -1, 1, -1, -1, -3, -1, -2, -1, -1, -1, -2, -1, -1, -1, -1, -2, -2, -2, -2, -1, -3, -1, -1, -2, -1, -1, -1, -2, 0, -1, -2, 0, -2, -1, -2, -1, -2, -2, -2, -1, -2, 0, -1, -1, -1, -1, -2, -1, -1, -1, -2, 0, -2, -1, -1, -1, -2, -3, -1, -2, -2, -1, -1, -2, -1, -1, -2, -1, -1, -2, -1, -1, -1, -2, -1, -2, -1, -2, -1, -2, -1, -1, -1, -1, -1, -2, -1, 0, -1, -1, -2, -1, -1, -2, -1, -1, -2, 1, -1, -2, -1, -1, -1, -2, -1, -2, -2, -1, -1, -2, 0, -1, -1, -2, -1, -1, -1, -2, -1, -2, -1, -2, -1, 0, -1, -1, -1, 0, -1, -1, -1, -1, -1, -1, -1, -2, -1, 0, -1, -1, -1, -1, -2, -1, -1, -2, -1, -1, -1, -1, -2, 0, -2, -1, -1, -2, -1, -1, -1, -1, -1, -1, -2, -1, -2, -1, -1, -1, -2, -1, -1, -1, -1, -1, -1, -1, -2, -2, -2, -1, -2, -1, -2, 0, -2, -1, -2, -2, -2, -1, -2, -2, -2, -1, -2, -1, -1, -1, -2, -2, -1, -2, -2, -2, 0, -1, -2, -1, -1, -1, -3, 1, -1, -2, -1, 0, -2, -1, -1, -1, -1, -1, -2, 2, -2, -1, -1, -2, -1, -2, -1, -1, -2, -1, -2, -1, 0, -2, -1, -2, -2, -1, -3, -1, -1, -1, -1, -1, -2, 1, -2, -2, -1, -1, 0, -2, 0, -1, -1, -2, -1, -2, -2, -1, -1, -2, -1, 0, -1, -1, -1, -1, -2, -2, -1, -1, -2, -2, -2, -1, -1, -1, -2, -1, -1, -2, -2, -1, -1, -2, -1, -1, -1, -1, -1, -1, -2, -2, -1, -2, -1, -2, 0, -1, -2, -2, -2, -1, -2, 1, -2, -2, -1, -1, -2, -1, -1, -1, -2, 0, -2, -1, -1, -1, -2, -1, -2, -1, -2, -1, -1, -2, 0, -1, -2, -1, -1, -1, -1, -1, -2, -1, -2, -1, -2, -1, -2, -2, -2, -1, -1, -1, -2, -1, 0, -1, -1, -1, -2, 0, -2, -1, -1, -1, -2, -2, -1, -2, -2, -1, -1, -1, -1, -1, -2, -2, -1, -2, -2, -1, -1, -1, -1, -2, -2, -2, -1, -2, -2, -1, -1, -2, -1, -1, -1, -1, -1, -2, -2, -1, -1, -2, -1, -1, -1, -1, -1, -1, -2, -1, -1, -1, -1, -2, -1, 0, -1, -1, 0, -1, -2, -2, -1, -1, -2, -1, -2, -1, 0, -1, -2, -2, -1, -1, -2, -1, -1, -2, -1, -1, -2, -1, -1, -1, -2, -1, -2, -2, -2, -1, -1, -1, -2, -1, -2, -1, -2, -2, -1, -1, -1, -1, -2, -1, -2, -1, -2, -2, -1, -1, -2, -1]
  in  "reset":i16[](array[numeric])
  out "toqueue":i32[][](array[numeric])
  out "time queue":i32[](array[numeric])
  out "data x queue":i32[](array[numeric])
  out "data y queue":i32[](array[numeric])
  out "?":string="this parameter determines how fast function reads data, higher value means slower reading and lower accuracy (use hundreds or thousands)"
  in  "ticks scope":u32=8500
  out "?":string="break count"
  in  "power threshold":i32=80
  in  "break count":u16=2
  in  "deviation precision":dbl=10.0
  in  "break length":u16=2
  in  "trigger ending mode":bool=TRUE
  out "?":string="break length"
  out "?":string="break count"
  out "trigger index":i32=799
  out "end trigger index":i32=710
  out "zero count break":u16
  out "end trigger":bool=TRUE
  in  "min/max precision":i16=6
  out "last":u16
  out "zero count lenght":u16
  in  "Filename template":path=path "C:/Users/User/Desktop/Tester_znakowarki/scope_template/template.lvm" caption="Filename"
  in  "Filename errors":path=path "C:/Users/User/Desktop/Tester_znakowarki/scope_errors/error.lvm" caption="Filename"
  in  "Filename history":path=path "C:/Users/User/Desktop/Tester_ znakowarki/scope_history/history.lvm" caption="Filename"
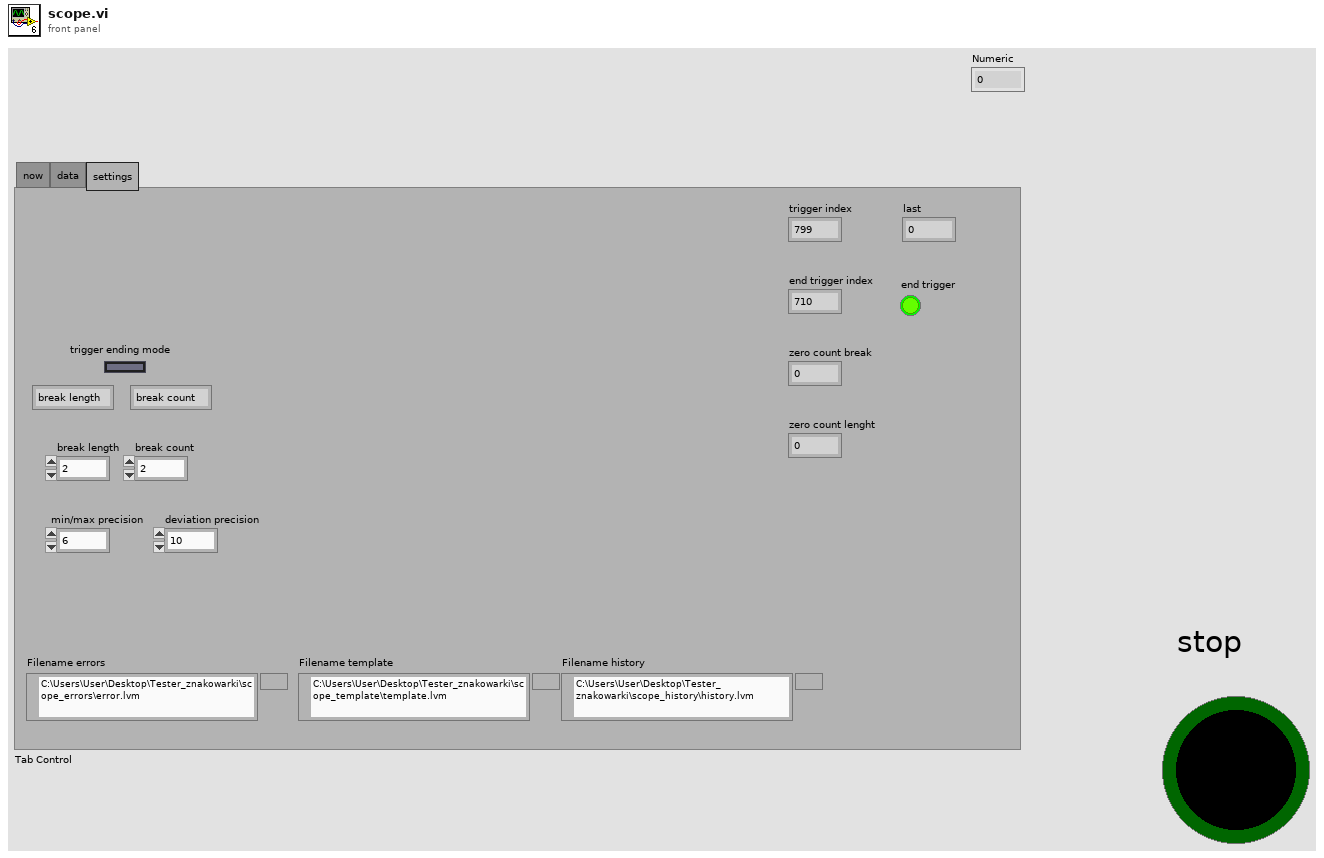
[diagram p1: front panel]
types:
  T1 = cluster{"time queue":i32[], "data x queue":i32[]}
  T2 = cluster{"time queue":i32[], "data y queue":i32[]}
  T3 = cluster{"time queue":i32[], "data y queue":i32[]}[]
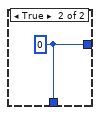
[diagram p2: hidden frame]
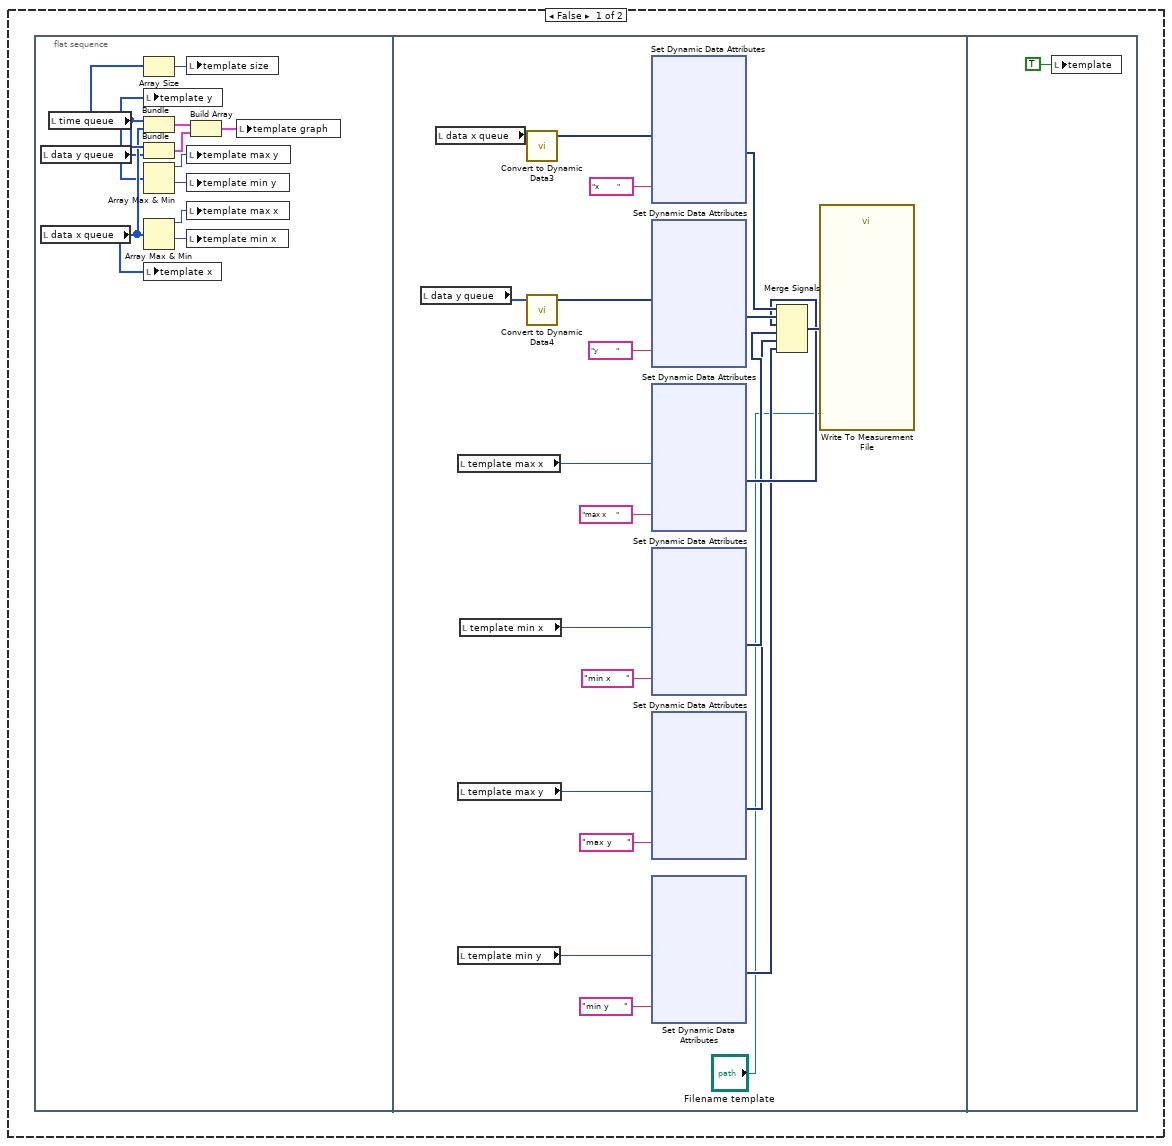
[diagram p3: hidden frame]
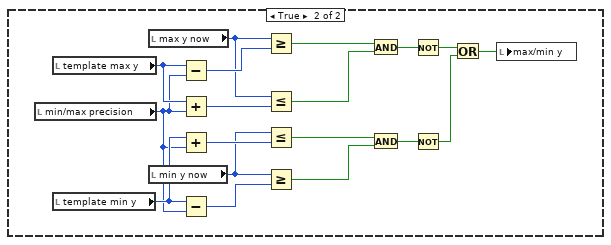
[diagram p4: hidden frame]
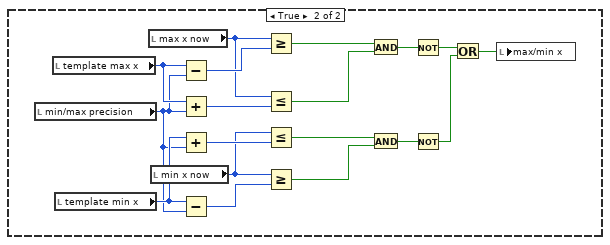
[diagram p5: hidden frame]
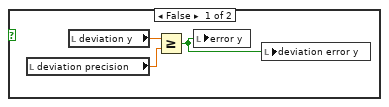
[diagram p6: hidden frame]
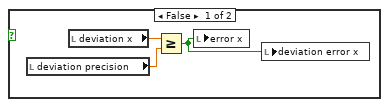
[diagram p7: hidden frame]
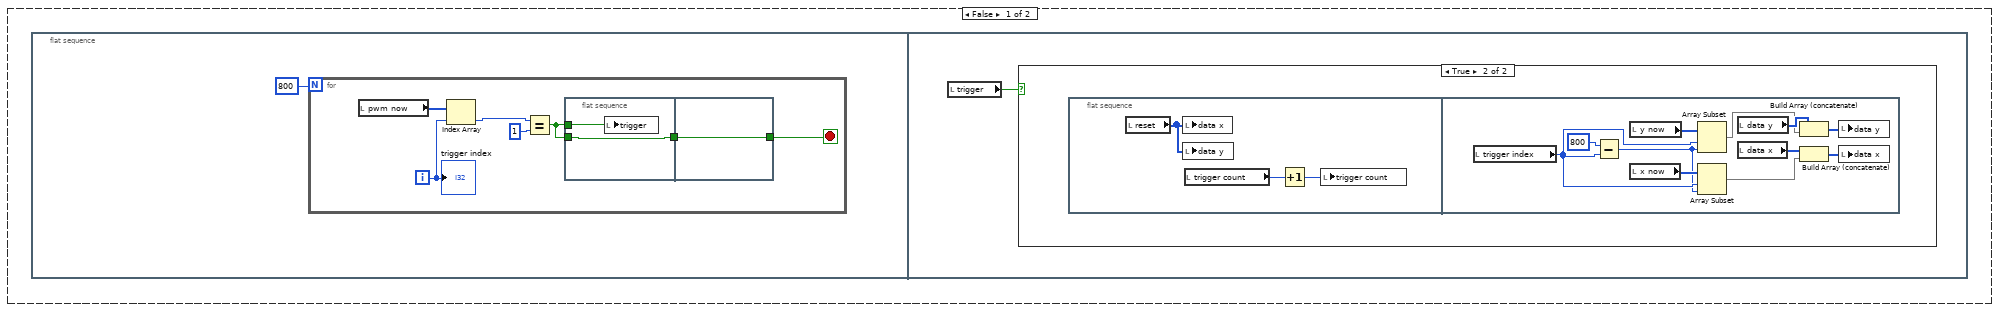
[diagram p9: hidden frame]
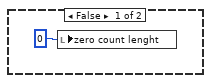
[diagram p11: hidden frame]
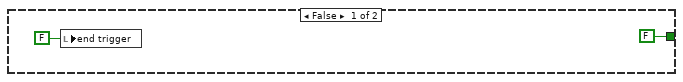
[diagram p12: hidden frame]
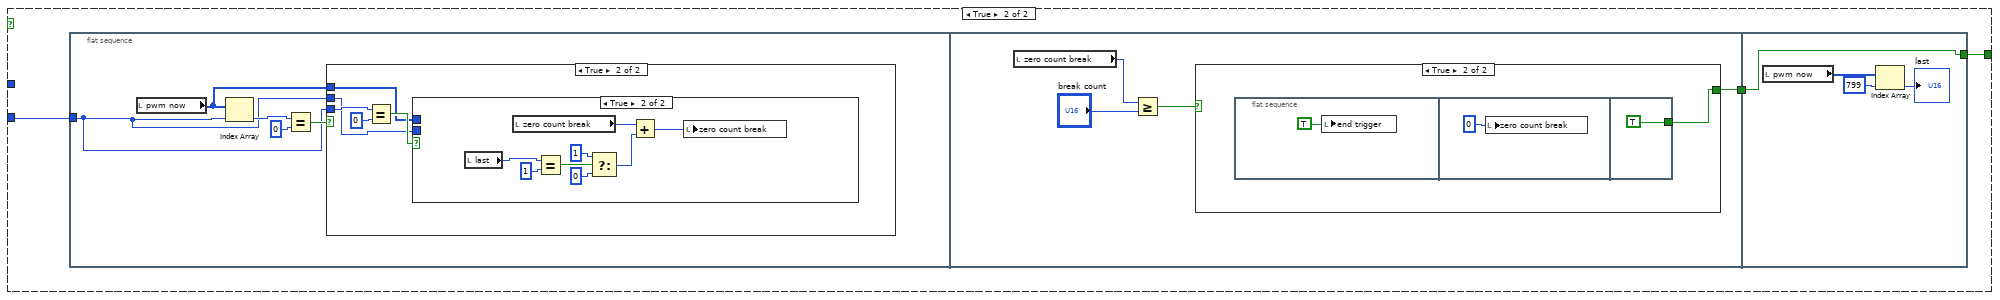
[diagram p13: hidden frame]
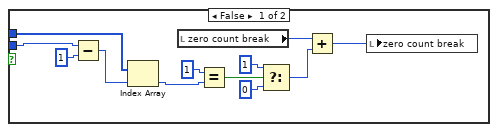
[diagram p15: hidden frame]
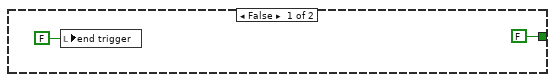
[diagram p16: hidden frame]
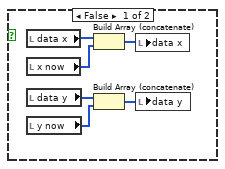
[diagram p17: hidden frame]
diagram:
  n1 = flat-sequence {
    tunnel: [w16] -> w8
    tunnel: [w15] -> w7
    frame #0 {
      w12 = FALSE ("error x now")
      w13 = u16 0 ("Numeric")
      n2 = local write "x now"("reset") -> ()
      n3 = local write "y now"("reset") -> ()
      n4 = local write "time"("reset") -> ()
      n5 = local write "data x"("reset") -> ()
      n6 = local write "data y"("reset") -> ()
      n7 = local write "stop"(w12) -> ()
      n8 = local write "pwm now"("reset") -> ()
      "trigger" <- w12
      "end trigger" <- w12
      "template" <- w12
      "zero count break" <- w13
      "max/min y" <- w12
      "max/min x" <- w12
      "error y" <- w12
      "error x" <- w12
      "size now" <- w13
      "template max x" <- w13
      "template min x" <- w13
      "template min y" <- w13
      "max x now" <- w13
      "min x now" <- w13
      "max y now" <- w13
      "min y now" <- w13
      "template size" <- w13
      "template max y" <- w13
      "trigger count" <- w13
      "deviation x" <- w13
      "deviation y" <- w13
      "deviation error y" <- w12
      "deviation error x" <- w12
      "zero count lenght" <- w13
    }
    frame #1 {
      n9 = xnode "Open FPGA VI Reference"("resource name"=tag "rio://172.22.11.2/RIO0") -> ("FPGA VI Reference Out"=w16:refnum<k20>, "error out"=w15:errorcluster)  [unwired: 1 in]
    }
  }
  n10 = xnode "Invoke Method"("FPGA VI Reference In"=w8, "error in"=w7, "Requested Depth"=u32 1024) -> ("FPGA VI Reference Out"=w6:refnum<k20>, "error out"=w5:errorcluster)  [unwired: 1 out]
  n11 = local read "trigger count"() -> (w4:i16)
  n12 = Obtain Queue(element data type=w4) -> (queue out=w1:refnum<queue>)  [unwired: 4 in, 2 out]
  n13 = local read "toqueue"() -> (w3:i32[][])
  n14 = Obtain Queue(element data type=w3) -> (queue out=w2:refnum<queue>)  [unwired: 4 in, 2 out]
  n15 = while {
    tunnel: w6 -> [w41]
    tunnel: w5 -> [w40]
    tunnel: [w33] -> w10
    tunnel: [w32] -> w9
    tunnel: w1 -> [w19]
    tunnel: w2 -> [w18]
    stop <- "stop" stop-if-true
    n16 = flat-sequence {
      frame #0 {
        n17 = local read "data x"() -> (w44:i16[])
        n18 = Array Size(array=w44) -> (size(s)=w43:i32)
        n19 = for {
          N: w43 -> [_]
          tunnel: [w45] -> w42 mode=indexing
          i -> [w45]
        }
        n20 = local write "time"(w42) -> ()
      }
      frame #1 {
        n21 = local read "data x"() -> (w47:i16[])
        n22 = local read "data y"() -> (w48:i16[])
        n23 = local read "time"() -> (w49:i32[])
        n24 = Bundle("time"=w49, "data x"=w47) -> (w50:cluster{"time":i32[], "data x":i16[]})  [unwired: 1 in]
        n25 = Bundle("time"=w49, "data y"=w48) -> (w51:cluster{"time":i32[], "data y":i16[]})  [unwired: 1 in]
        n26 = Build Array(w50, w51) -> (w46:cluster{"time":i32[], "data y":i16[]}[])
        n27 = local write "data graph"(w46) -> ()
      }
    }
    n28 = local read "trigger"() -> (w21:bool)
    n29 = case shown="True" w21 {
      tunnel: w18 -> [_ w79]
      tunnel: w19 -> [_ w78]
      frame False {
        n30 = flat-sequence {
          frame #0 {
            n31 = for {
              N: 800 -> [_]
              i -> [w58]
              stop <- w53 stop-if-true
              n32 = local read "pwm now"() -> (w59:u16[])
              n33 = Index Array(array=w59, index=w58) -> (element=w57:u16)
              n34 = Equal?(x=w57, y=u16 1) -> (x = y?=w54:bool)
              n35 = flat-sequence {
                tunnel: w54 -> [w61]
                tunnel: [w60] -> w55
                tunnel: w54 -> [w60]
                tunnel: w55 -> [w62]
                tunnel: [w62] -> w53
                frame #0 {
                  n36 = local write "trigger"(w61) -> ()
                }
                frame #1 {
                }
              }
              "trigger index" <- w58
            }
          }
          frame #1 {
            n37 = local read "trigger"() -> (w63:bool)
            n38 = case shown="True" w63 {
              frame False {
              }
              frame True {
                n39 = flat-sequence {
                  frame #0 {
                    n40 = local read "reset"() -> (w66:i16[])
                    n41 = local write "data x"(w66) -> ()
                    n42 = local write "data y"(w66) -> ()
                    n43 = local read "trigger count"() -> (w65:i16)
                    n44 = Increment(x=w65) -> (x+1=w64:i16)
                    n45 = local write "trigger count"(w64) -> ()
                  }
                  frame #1 {
                    n46 = local read "trigger index"() -> (w75:i32)
                    n47 = Subtract(x=800, y=w75) -> (x-y=w73:i32)
                    n48 = local read "y now"() -> (w74:i16[])
                    n49 = local read "x now"() -> (w76:i16[])
                    n50 = Array Subset(array=w74, index=w75, length=w73) -> (w70:i16[])
                    n51 = Array Subset(array=w76, index=w75, length=w73) -> (w69:i16[])
                    n52 = local read "data y"() -> (w72:i16[])
                    n53 = local read "data x"() -> (w68:i16[])
                    n54 = Build Array (concatenate)(w72, w70) -> (w71:i16[])
                    n55 = Build Array (concatenate)(w68, w69) -> (w67:i16[])
                    n56 = local write "data y"(w71) -> ()
                    n57 = local write "data x"(w67) -> ()
                  }
                }
              }
            }
          }
        }
      }
      frame True {
        n58 = flat-sequence {
          tunnel: w79 -> [w153]
          tunnel: w78 -> [w152]
          frame #0 {
            n59 = for {
              N: 800 -> [_]
              i -> [w81]
              stop <- w83 stop-if-true
              n60 = case shown="False" "trigger ending mode" {
                tunnel: [w84 w106] -> w83
                tunnel: w81 -> [_ w105]
                tunnel: w81 -> [w85 _]
                frame False {
                  n61 = flat-sequence {
                    tunnel: w85 -> [w89]
                    tunnel: [w95] -> w84
                    frame #0 {
                      n62 = local read "pwm now"() -> (w90:u16[])
                      n63 = Index Array(array=w90, index=w89) -> (element=w88:u16)
                      n64 = Equal?(x=w88, y=u16 0) -> (x = y?=w86:bool)
                      n65 = case shown="True" w86 {
                        frame False {
                          n66 = local write "zero count lenght"(u16 0 ("zero count 2")) -> ()
                        }
                        frame True {
                          n67 = local read "zero count lenght"() -> (w93:u16)
                          n68 = Add(x=w93, y=u16 1) -> (x+y=w94:u16)
                          n69 = local write "zero count lenght"(w94) -> ()
                        }
                      }
                    }
                    frame #1 {
                      n70 = local read "zero count lenght"() -> (w98:u16)
                      n71 = Greater Or Equal?(x=w98, y="break length") -> (x >= y?=w96:bool)
                      n72 = case shown="True" w96 {
                        tunnel: [FALSE w101] -> w95
                        frame False {
                          n73 = local write "end trigger"(FALSE ("end trigger")) -> ()
                        }
                        frame True {
                          n74 = flat-sequence {
                            tunnel: [TRUE] -> w101
                            frame #0 {
                              n75 = local write "end trigger"(TRUE ("end trigger")) -> ()
                            }
                            frame #1 {
                              n76 = local write "zero count lenght"(u16 0 ("zero count 2")) -> ()
                            }
                            frame #2 {
                            }
                          }
                        }
                      }
                    }
                  }
                }
                frame True {
                  n77 = flat-sequence {
                    tunnel: w105 -> [w109]
                    tunnel: [w138] -> w107
                    tunnel: [w151] -> w106
                    tunnel: w107 -> [w151]
                    frame #0 {
                      n78 = local read "pwm now"() -> (w108:u16[])
                      n79 = Index Array(array=w108, index=w109) -> (element=w112:u16)
                      n80 = Equal?(x=w112, y=u16 0) -> (x = y?=w110:bool)
                      n81 = case shown="True" w110 {
                        tunnel: w109 -> [_ w117]
                        tunnel: w109 -> [_ w114]
                        tunnel: w108 -> [_ w113]
                        frame False {
                        }
                        frame True {
                          n82 = Equal?(x=w117, y=0) -> (x = y?=w115:bool)
                          n83 = case shown="True" w115 {
                            tunnel: w114 -> [w129 _]
                            tunnel: w113 -> [w126 _]
                            frame False {
                              n84 = Subtract(x=w129, y=1) -> (x-y=w127:i32)
                              n85 = Index Array(array=w126, index=w127) -> (element=w125:u16)
                              n86 = local read "zero count break"() -> (w119:u16)
                              n87 = Equal?(x=u16 1, y=w125) -> (x = y?=w123:bool)
                              n88 = Select(t=i16 1, s=w123, f=i16 0) -> (s? t:f=w120:i16)
                              n89 = Add(x=w119, y=w120) -> (x+y=w118:u16)
                              n90 = local write "zero count break"(w118) -> ()
                            }
                            frame True {
                              n91 = local read "last"() -> (w137:u16)
                              n92 = local read "zero count break"() -> (w131:u16)
                              n93 = Equal?(x=w137, y=u16 1) -> (x = y?=w135:bool)
                              n94 = Select(t=i16 1, s=w135, f=i16 0) -> (s? t:f=w130:i16)
                              n95 = Add(x=w131, y=w130) -> (x+y=w132:u16)
                              n96 = local write "zero count break"(w132) -> ()
                            }
                          }
                        }
                      }
                    }
                    frame #1 {
                      n97 = local read "zero count break"() -> (w139:u16)
                      n98 = Greater Or Equal?(x=w139, y="break count") -> (x >= y?=w141:bool)
                      n99 = case shown="True" w141 {
                        tunnel: [FALSE w144] -> w138
                        frame False {
                          n100 = local write "end trigger"(FALSE ("end trigger")) -> ()
                        }
                        frame True {
                          n101 = flat-sequence {
                            tunnel: [TRUE] -> w144
                            frame #0 {
                              n102 = local write "end trigger"(TRUE ("mini trigger")) -> ()
                            }
                            frame #1 {
                              n103 = local write "zero count break"(u16 0 ("zero count")) -> ()
                            }
                            frame #2 {
                            }
                          }
                        }
                      }
                    }
                    frame #2 {
                      n104 = local read "pwm now"() -> (w150:u16[])
                      n105 = Index Array(array=w150, index=799) -> (element=→"last":u16)
                    }
                  }
                }
              }
              "end trigger index" <- w81
            }
          }
          frame #1 {
            n106 = local read "end trigger"() -> (w154:bool)
            n107 = case shown="True" w154 {
              tunnel: w153 -> [_ w162]
              tunnel: w152 -> [_ w161]
              frame False {
                n108 = local read "data x"() -> (w159:i16[])
                n109 = local read "x now"() -> (w160:i16[])
                n110 = local read "data y"() -> (w156:i16[])
                n111 = local read "y now"() -> (w155:i16[])
                n112 = Build Array (concatenate)(w159, w160) -> (w158:i16[])
                n113 = Build Array (concatenate)(w156, w155) -> (w157:i16[])
                n114 = local write "data x"(w158) -> ()
                n115 = local write "data y"(w157) -> ()
              }
              frame True {
                n116 = flat-sequence {
                  tunnel: w162 -> [w187]
                  tunnel: w161 -> [w184]
                  frame #0 {
                    w171 = 0 ("index")
                    n117 = local read "end trigger index"() -> (w172:i32)
                    n118 = local read "y now"() -> (w170:i16[])
                    n119 = local read "x now"() -> (w169:i16[])
                    n120 = Array Subset(array=w170, index=w171, length=w172) -> (w167:i16[])
                    n121 = Array Subset(array=w169, index=w171, length=w172) -> (w168:i16[])
                    n122 = local read "data y"() -> (w166:i16[])
                    n123 = local read "data x"() -> (w165:i16[])
                    n124 = Build Array (concatenate)(w166, w167) -> (w164:i16[])
                    n125 = Build Array (concatenate)(w165, w168) -> (w163:i16[])
                    n126 = local write "data y"(w164) -> ()
                    n127 = local write "data x"(w163) -> ()
                  }
                  frame #1 {
                    n128 = local read "data x"() -> (w175:i16[])
                    n129 = Array Size(array=w175) -> (size(s)=w174:i32)
                    n130 = for {
                      N: w174 -> [_]
                      tunnel: [w176] -> w173 mode=indexing
                      i -> [w176]
                    }
                    n131 = local write "time"(w173) -> ()
                  }
                  frame #2 {
                    n132 = local read "data x"() -> (w180:i16[])
                    n133 = local read "data y"() -> (w181:i16[])
                    n134 = local read "time"() -> (w182:i32[])
                    n135 = local write "trigger"(FALSE ("end trigger")) -> ()
                    n136 = Bundle("time"=w182, "data x"=w180) -> (w179:cluster{"time":i32[], "data x":i16[]})  [unwired: 1 in]
                    n137 = Bundle("time"=w182, "data y"=w181) -> (w178:cluster{"time":i32[], "data y":i16[]})  [unwired: 1 in]
                    n138 = Build Array(w179, w178) -> (w177:cluster{"time":i32[], "data y":i16[]}[])
                    n139 = local write "data graph"(w177) -> ()
                  }
                  frame #3 {
                    n140 = local read "time"() -> (w190:i32[])
                    n141 = local read "data x"() -> (w189:i16[])
                    n142 = local read "data y"() -> (w188:i16[])
                    n143 = local read "trigger count"() -> (w185:i16)
                    n144 = Build Array(w190, w189, w188) -> (w186:i32[][])
                    "toqueue" <- w186
                    n145 = Enqueue Element(queue=w184, element=w185) -> ()  [unwired: 2 in, 3 out]
                    n146 = Enqueue Element(queue=w187, element=w186) -> ()  [unwired: 2 in, 3 out]
                  }
                  frame #4 {
                    n147 = local read "end trigger index"() -> (w191:i32)
                    n148 = local read "pwm now"() -> (w194:u16[])
                    n149 = Subtract(x=800, y=w191) -> (x-y=w193:i32)
                    n150 = Array Subset(array=w194, index=w191, length=w193) -> (w192:u16[])
                    n151 = for {
                      N: w193 -> [_]
                      tunnel: w192 -> [w204]
                      tunnel: w191 -> [w198]
                      i -> [w197]
                      stop <- w199 stop-if-true
                      n152 = Add(x=w198, y=w197) -> (x+y=w196:i32)
                      n153 = Index Array(array=w204, index=w197) -> (element=w203:u16)
                      n154 = local write "trigger index"(w196) -> ()
                      n155 = Equal?(x=w203, y=u16 1) -> (x = y?=w200:bool)
                      n156 = flat-sequence {
                        tunnel: w200 -> [w206]
                        tunnel: [w205] -> w201
                        tunnel: w200 -> [w205]
                        tunnel: w201 -> [w207]
                        tunnel: [w207] -> w199
                        frame #0 {
                          n157 = local write "trigger"(w206) -> ()
                        }
                        frame #1 {
                        }
                      }
                    }
                  }
                  frame #5 {
                    n158 = local read "trigger"() -> (w208:bool)
                    n159 = case shown="True" w208 {
                      frame False {
                      }
                      frame True {
                        n160 = flat-sequence {
                          frame #0 {
                            n161 = local read "reset"() -> (w211:i16[])
                            n162 = local read "trigger count"() -> (w210:i16)
                            n163 = local write "data x"(w211) -> ()
                            n164 = local write "data y"(w211) -> ()
                            n165 = Increment(x=w210) -> (x+1=w209:i16)
                            n166 = local write "trigger count"(w209) -> ()
                          }
                          frame #1 {
                            n167 = local read "trigger index"() -> (w212:i32)
                            n168 = Subtract(x=800, y=w212) -> (x-y=w213:i32)
                            n169 = local read "x now"() -> (w222:i16[])
                            n170 = local read "y now"() -> (w221:i16[])
                            n171 = Array Subset(array=w222, index=w212, length=w213) -> (w215:i16[])
                            n172 = Array Subset(array=w221, index=w212, length=w213) -> (w216:i16[])
                            n173 = local read "data x"() -> (w220:i16[])
                            n174 = local read "data y"() -> (w219:i16[])
                            n175 = Build Array (concatenate)(w220, w215) -> (w218:i16[])
                            n176 = Build Array (concatenate)(w219, w216) -> (w217:i16[])
                            n177 = local write "data x"(w218) -> ()
                            n178 = local write "data y"(w217) -> ()
                          }
                        }
                      }
                    }
                  }
                }
              }
            }
          }
        }
      }
    }
    n179 = xnode "Read/Write Control"("FPGA VI Reference In"=w41, "error in"=w40, "count ticks scope"="ticks scope") -> ("FPGA VI Reference Out"=w39:refnum<k20>, "error out"=w38:errorcluster)
    n180 = xnode "Read/Write Control"("FPGA VI Reference In"=w39, "error in"=w38, "power threshold (scope)"="power threshold") -> ("FPGA VI Reference Out"=w35:refnum<k20>, "error out"=w34:errorcluster)
    n181 = xnode "Invoke Method"("FPGA VI Reference In"=w35, "error in"=w34, "Number of Elements"=u32 800, "Timeout (ms)"=-1) -> ("FPGA VI Reference Out"=w33:refnum<k20>, "error out"=w32:errorcluster, "Data"=w29:u64[])  [unwired: 1 out]
    n182 = Split Number(x=w29) -> (hi(x)=w28:u32[], lo(x)=w27:u32[])
    n183 = Split Number(x=w28) -> (hi(x)=→"pwm now":u16[])  [unwired: 1 out]
    n184 = Split Number(x=w27) -> (hi(x)=w26:u16[], lo(x)=w25:u16[])
    n185 = To Word Integer(number=w26) -> (16bit integer=→"x now":i16[])
    n186 = To Word Integer(number=w25) -> (16bit integer=→"y now":i16[])
  }
  n187 = while {
    tunnel: w2 -> [w224]
    tunnel: w1 -> [w225]
    i -> [w223]
    stop <- w226 stop-if-true
    n188 = flat-sequence {
      tunnel: w225 -> [w228]
      tunnel: w224 -> [w227]
      frame #0 {
        n189 = flat-sequence {
          tunnel: w228 -> [w233]
          tunnel: w227 -> [w232]
          frame #0 {
            n190 = local read "stop"() -> (w231:bool)
            n191 = case shown="False" w231 {
              tunnel: [w236 w237] -> w230
              tunnel: [w236 w237] -> w229
              frame False {
                w236 = -1
              }
              frame True {
                w237 = 0
              }
            }
            n192 = Dequeue Element(queue=w232, timeout in ms (-1)=w229) -> (element=→"inqueue":i32[][])  [unwired: 1 in, 3 out]
            n193 = Dequeue Element(queue=w233, timeout in ms (-1)=w230) -> (element=→"trigger count queue":i16)  [unwired: 1 in, 3 out]
          }
          frame #1 {
            n194 = local read "inqueue"() -> (w244:i32[][])
            n195 = local read "inqueue"() -> (w243:i32[][])
            n196 = local read "inqueue"() -> (w241:i32[][])
            n197 = Index Array(array=w244, index (row)=2) -> (element=→"data y queue":i32[])  [unwired: 1 in]
            n198 = Index Array(array=w241, index (row)=0) -> (element=→"time queue":i32[])  [unwired: 1 in]
            n199 = Index Array(array=w243, index (row)=1) -> (element=→"data x queue":i32[])  [unwired: 1 in]
          }
        }
      }
      frame #1 {
        n200 = local read "template"() -> (w247:bool)
        n201 = case shown="True" w247 {
          frame False {
            n202 = flat-sequence {
              frame #0 {
                n203 = local read "data y queue"() -> (w248:i32[])
                n204 = local read "data x queue"() -> (w249:i32[])
                n205 = local read "time queue"() -> (w255:i32[])
                n206 = Array Size(array=w255) -> (size(s)=w254:i32)
                n207 = local write "template y"(w248) -> ()
                n208 = Bundle("time queue"=w255, "data x queue"=w249) -> (w258:T1)  [unwired: 1 in]
                n209 = Bundle("time queue"=w255, "data y queue"=w248) -> (w257:T2)  [unwired: 1 in]
                n210 = Array Max & Min(array=w248) -> (max value=w251:i32, min value=w250:i32)  [unwired: 2 out]
                n211 = Array Max & Min(array=w249) -> (max value=w253:i32, min value=w252:i32)  [unwired: 2 out]
                n212 = local write "template x"(w249) -> ()
                n213 = local write "template size"(w254) -> ()
                n214 = local write "template max y"(w251) -> ()
                n215 = local write "template min y"(w250) -> ()
                n216 = local write "template max x"(w253) -> ()
                n217 = local write "template min x"(w252) -> ()
                n218 = Build Array(w258, w257) -> (w256:T3)
                n219 = local write "template graph"(w256) -> ()
              }
              frame #1 {
                n220 = local read "data y queue"() -> (w277:i32[])
                n221 = local read "data x queue"() -> (w279:i32[])
                n222 = local read "template max x"() -> (w273:i16)
                n223 = local read "template max y"() -> (w268:i16)
                n224 = local read "template min y"() -> (w267:i16)
                n225 = local read "template min x"() -> (w271:i16)
                n226 = call "Convert to Dynamic Data3"("Array"=w279) -> ("Dynamic Data Type"=w278:dynamicdata)  [unwired: 3 in]
                n227 = call "Convert to Dynamic Data4"("Array"=w277) -> ("Dynamic Data Type"=w276:dynamicdata)  [unwired: 3 in]
                n228 = xnode "Set Dynamic Data Attributes"("Signals In"=w278, "Signal Name"="x         ") -> ("Signals Out"=w274:dynamicdata)  [unwired: 2 in, 1 out]
                n229 = xnode "Set Dynamic Data Attributes"("Signals In"=w276, "Signal Name"="y         ") -> ("Signals Out"=w275:dynamicdata)  [unwired: 2 in, 1 out]
                n230 = xnode "Set Dynamic Data Attributes"("Signals In"=w273, "Signal Name"="max x     ") -> ("Signals Out"=w272:dynamicdata)  [unwired: 2 in, 1 out]
                n231 = xnode "Set Dynamic Data Attributes"("Signals In"=w271, "Signal Name"="min x     ") -> ("Signals Out"=w270:dynamicdata)  [unwired: 2 in, 1 out]
                n232 = xnode "Set Dynamic Data Attributes"("Signals In"=w268, "Signal Name"="max y     ") -> ("Signals Out"=w269:dynamicdata)  [unwired: 2 in, 1 out]
                n233 = xnode "Set Dynamic Data Attributes"("Signals In"=w267, "Signal Name"="min y     ") -> ("Signals Out"=w266:dynamicdata)  [unwired: 2 in, 1 out]
                n234 = Merge Signals(w274, w275, w272, w270, w269, w266) -> (w280:dynamicdata)
                n235 = call "Write To Measurement File"("Signals"=w280, "Filename"="Filename template") -> ()  [unwired: 15 in, 3 out]
              }
              frame #2 {
                n236 = local write "template"(TRUE ("template")) -> ()
              }
            }
          }
          frame True {
            n237 = flat-sequence {
              frame #0 {
                n238 = local read "data x queue"() -> (w373:i32[])
                n239 = local read "data y queue"() -> (w372:i32[])
                n240 = local read "time queue"() -> (w366:i32[])
                n241 = Array Size(array=w366) -> (size(s)=w367:i32)
                n242 = Array Max & Min(array=w373) -> (max value=w371:i32, min value=w370:i32)  [unwired: 2 out]
                n243 = Array Max & Min(array=w372) -> (max value=w369:i32, min value=w368:i32)  [unwired: 2 out]
                n244 = local write "size now"(w367) -> ()
                n245 = local write "max x now"(w371) -> ()
                n246 = local write "min x now"(w370) -> ()
                n247 = local write "max y now"(w369) -> ()
                n248 = local write "min y now"(w368) -> ()
              }
              frame #1 {
                n249 = local read "error x"() -> (w374:bool)
                n250 = local read "error y"() -> (w375:bool)
                n251 = case shown="False" w374 {
                  frame False {
                    n252 = local read "min/max precision"() -> (w415:i16)
                    n253 = local read "template max x"() -> (w417:i16)
                    n254 = local read "template min x"() -> (w416:i16)
                    n255 = local read "max x now"() -> (w418:i16)
                    n256 = local read "min x now"() -> (w419:i16)
                    n257 = Subtract(x=w417, y=w415) -> (x-y=w422:i16)
                    n258 = Add(x=w417, y=w415) -> (x+y=w423:i16)
                    n259 = Add(x=w416, y=w415) -> (x+y=w421:i16)
                    n260 = Subtract(x=w416, y=w415) -> (x-y=w420:i16)
                    n261 = Greater Or Equal?(x=w418, y=w422) -> (x >= y?=w429:bool)
                    n262 = Less Or Equal?(x=w418, y=w423) -> (x <= y?=w428:bool)
                    n263 = Less Or Equal?(x=w419, y=w421) -> (x <= y?=w426:bool)
                    n264 = Greater Or Equal?(x=w419, y=w420) -> (x >= y?=w425:bool)
                    n265 = And(x=w429, y=w428) -> (x .and. y?=w427:bool)
                    n266 = And(x=w426, y=w425) -> (x .and. y?=w424:bool)
                    n267 = Not(x=w427) -> (.not. x?=w413:bool)
                    n268 = Not(x=w424) -> (.not. x?=w414:bool)
                    n269 = Or(x=w413, y=w414) -> (x .or. y?=w412:bool)
                    n270 = local write "error x"(w412) -> ()
                    n271 = local write "max/min x"(w412) -> ()
                  }
                  frame True {
                    n272 = local read "min/max precision"() -> (w430:i16)
                    n273 = local read "template max x"() -> (w434:i16)
                    n274 = local read "template min x"() -> (w432:i16)
                    n275 = local read "max x now"() -> (w433:i16)
                    n276 = local read "min x now"() -> (w431:i16)
                    n277 = Subtract(x=w434, y=w430) -> (x-y=w440:i16)
                    n278 = Add(x=w434, y=w430) -> (x+y=w441:i16)
                    n279 = Add(x=w432, y=w430) -> (x+y=w439:i16)
                    n280 = Subtract(x=w432, y=w430) -> (x-y=w438:i16)
                    n281 = Greater Or Equal?(x=w433, y=w440) -> (x >= y?=w447:bool)
                    n282 = Less Or Equal?(x=w433, y=w441) -> (x <= y?=w446:bool)
                    n283 = Less Or Equal?(x=w431, y=w439) -> (x <= y?=w444:bool)
                    n284 = Greater Or Equal?(x=w431, y=w438) -> (x >= y?=w443:bool)
                    n285 = And(x=w447, y=w446) -> (x .and. y?=w445:bool)
                    n286 = And(x=w444, y=w443) -> (x .and. y?=w442:bool)
                    n287 = Not(x=w445) -> (.not. x?=w436:bool)
                    n288 = Not(x=w442) -> (.not. x?=w437:bool)
                    n289 = Or(x=w436, y=w437) -> (x .or. y?=w435:bool)
                    n290 = local write "max/min x"(w435) -> ()
                  }
                }
                n291 = case shown="False" w375 {
                  frame False {
                    n292 = local read "min/max precision"() -> (w377:i16)
                    n293 = local read "template max y"() -> (w381:i16)
                    n294 = local read "template min y"() -> (w379:i16)
                    n295 = local read "max y now"() -> (w380:i16)
                    n296 = local read "min y now"() -> (w378:i16)
                    n297 = Subtract(x=w381, y=w377) -> (x-y=w386:i16)
                    n298 = Add(x=w381, y=w377) -> (x+y=w387:i16)
                    n299 = Add(x=w379, y=w377) -> (x+y=w385:i16)
                    n300 = Subtract(x=w379, y=w377) -> (x-y=w384:i16)
                    n301 = Greater Or Equal?(x=w380, y=w386) -> (x >= y?=w393:bool)
                    n302 = Less Or Equal?(x=w380, y=w387) -> (x <= y?=w392:bool)
                    n303 = Less Or Equal?(x=w378, y=w385) -> (x <= y?=w390:bool)
                    n304 = Greater Or Equal?(x=w378, y=w384) -> (x >= y?=w389:bool)
                    n305 = And(x=w393, y=w392) -> (x .and. y?=w391:bool)
                    n306 = And(x=w390, y=w389) -> (x .and. y?=w388:bool)
                    n307 = Not(x=w391) -> (.not. x?=w383:bool)
                    n308 = Not(x=w388) -> (.not. x?=w382:bool)
                    n309 = Or(x=w383, y=w382) -> (x .or. y?=w376:bool)
                    n310 = local write "error y"(w376) -> ()
                    n311 = local write "max/min y"(w376) -> ()
                  }
                  frame True {
                    n312 = local read "min/max precision"() -> (w397:i16)
                    n313 = local read "template max y"() -> (w399:i16)
                    n314 = local read "template min y"() -> (w398:i16)
                    n315 = local read "max y now"() -> (w401:i16)
                    n316 = local read "min y now"() -> (w400:i16)
                    n317 = Subtract(x=w399, y=w397) -> (x-y=w404:i16)
                    n318 = Add(x=w399, y=w397) -> (x+y=w405:i16)
                    n319 = Add(x=w398, y=w397) -> (x+y=w403:i16)
                    n320 = Subtract(x=w398, y=w397) -> (x-y=w402:i16)
                    n321 = Greater Or Equal?(x=w401, y=w404) -> (x >= y?=w411:bool)
                    n322 = Less Or Equal?(x=w401, y=w405) -> (x <= y?=w410:bool)
                    n323 = Less Or Equal?(x=w400, y=w403) -> (x <= y?=w408:bool)
                    n324 = Greater Or Equal?(x=w400, y=w402) -> (x >= y?=w407:bool)
                    n325 = And(x=w411, y=w410) -> (x .and. y?=w409:bool)
                    n326 = And(x=w408, y=w407) -> (x .and. y?=w406:bool)
                    n327 = Not(x=w409) -> (.not. x?=w396:bool)
                    n328 = Not(x=w406) -> (.not. x?=w395:bool)
                    n329 = Or(x=w396, y=w395) -> (x .or. y?=w394:bool)
                    n330 = local write "max/min y"(w394) -> ()
                  }
                }
              }
              frame #2 {
                n331 = local write "deviation y"(0.0 ("deviation y")) -> ()
                n332 = local write "deviation x"(0.0 ("deviation x")) -> ()
              }
              frame #3 {
                n333 = local read "template x"() -> (w455:i16[])
                n334 = local read "template y"() -> (w451:i16[])
                n335 = local read "data x queue"() -> (w457:i32[])
                n336 = local read "data y queue"() -> (w450:i32[])
                n337 = Array Size(array=w457) -> (size(s)=w459:i32)
                n338 = Array Size(array=w455) -> (size(s)=w458:i32)
                n339 = Array Size(array=w450) -> (size(s)=w453:i32)
                n340 = Array Size(array=w451) -> (size(s)=w452:i32)
                n341 = Max & Min(x=w459, y=w458) -> (min(x,y)=w456:i32)  [unwired: 1 out]
                n342 = Max & Min(x=w453, y=w452) -> (min(x,y)=w454:i32)  [unwired: 1 out]
                n343 = for {
                  N: w456 -> [w477]
                  tunnel: w455 -> [w483]
                  tunnel: w457 -> [w482]
                  i -> [w481]
                  n344 = Index Array(array=w482, index=w481) -> (element=w480:i32)
                  n345 = Index Array(array=w483, index=w481) -> (element=w479:i16)
                  n346 = Subtract(x=w480, y=w479) -> (x-y=w473:i32)
                  n347 = To Long Integer(number=w473) -> (32bit integer=w472:i32)
                  n348 = Square(x=w472) -> (x^2=w476:i32)
                  n349 = local read "deviation x"() -> (w474:dbl)
                  n350 = Divide(x=w476, y=w477) -> (x/y=w475:dbl)
                  n351 = Add(x=w475, y=w474) -> (x+y=w478:dbl)
                  n352 = local write "deviation x"(w478) -> ()
                }
                n353 = for {
                  N: w454 -> [w469]
                  tunnel: w451 -> [w468]
                  tunnel: w450 -> [w467]
                  i -> [w464]
                  n354 = Index Array(array=w467, index=w464) -> (element=w466:i32)
                  n355 = Index Array(array=w468, index=w464) -> (element=w465:i16)
                  n356 = Subtract(x=w466, y=w465) -> (x-y=w461:i32)
                  n357 = To Long Integer(number=w461) -> (32bit integer=w460:i32)
                  n358 = Square(x=w460) -> (x^2=w471:i32)
                  n359 = local read "deviation y"() -> (w463:dbl)
                  n360 = Divide(x=w471, y=w469) -> (x/y=w470:dbl)
                  n361 = Add(x=w470, y=w463) -> (x+y=w462:dbl)
                  n362 = local write "deviation y"(w462) -> ()
                }
              }
              frame #4 {
                n363 = local read "error x"() -> (w484:bool)
                n364 = local read "error y"() -> (w485:bool)
                n365 = case shown="True" w484 {
                  frame False {
                    n366 = local read "deviation precision"() -> (w493:dbl)
                    n367 = local read "deviation x"() -> (w494:dbl)
                    n368 = Greater Or Equal?(x=w494, y=w493) -> (x >= y?=w492:bool)
                    n369 = local write "error x"(w492) -> ()
                    n370 = local write "deviation error x"(w492) -> ()
                  }
                  frame True {
                    n371 = local read "deviation precision"() -> (w497:dbl)
                    n372 = local read "deviation x"() -> (w496:dbl)
                    n373 = Greater Or Equal?(x=w496, y=w497) -> (x >= y?=w495:bool)
                    n374 = local write "deviation error x"(w495) -> ()
                  }
                }
                n375 = case shown="True" w485 {
                  frame False {
                    n376 = local read "deviation precision"() -> (w487:dbl)
                    n377 = local read "deviation y"() -> (w488:dbl)
                    n378 = Greater Or Equal?(x=w488, y=w487) -> (x >= y?=w486:bool)
                    n379 = local write "error y"(w486) -> ()
                    n380 = local write "deviation error y"(w486) -> ()
                  }
                  frame True {
                    n381 = local read "deviation precision"() -> (w491:dbl)
                    n382 = local read "deviation y"() -> (w490:dbl)
                    n383 = Greater Or Equal?(x=w490, y=w491) -> (x >= y?=w489:bool)
                    n384 = local write "deviation error y"(w489) -> ()
                  }
                }
              }
              frame #5 {
                n385 = local read "deviation error y"() -> (w501:bool)
                n386 = local read "deviation error x"() -> (w502:bool)
                n387 = local read "max/min x"() -> (w503:bool)
                n388 = local read "max/min y"() -> (w504:bool)
                n389 = Or(x=w503, y=w504) -> (x .or. y?=w499:bool)
                n390 = Or(x=w502, y=w501) -> (x .or. y?=w500:bool)
                n391 = Or(x=w499, y=w500) -> (x .or. y?=w498:bool)
                n392 = case shown="True" w498 {
                  frame False {
                  }
                  frame True {
                    n393 = local read "data x queue"() -> (w526:i32[])
                    n394 = local read "data y queue"() -> (w525:i32[])
                    n395 = local read "max x now"() -> (w519:i16)
                    n396 = local read "max y now"() -> (w517:i16)
                    n397 = local read "min y now"() -> (w516:i16)
                    n398 = local read "min x now"() -> (w518:i16)
                    n399 = local read "trigger count queue"() -> (w522:i16)
                    n400 = call "Convert to Dynamic Data"("Array"=w526) -> ("Dynamic Data Type"=w534:dynamicdata)  [unwired: 3 in]
                    n401 = call "Convert to Dynamic Data2"("Array"=w525) -> ("Dynamic Data Type"=w533:dynamicdata)  [unwired: 3 in]
                    n402 = local read "deviation y"() -> (w521:dbl)
                    n403 = local read "deviation x"() -> (w520:dbl)
                    n404 = xnode "Set Dynamic Data Attributes"("Signals In"=w534, "Signal Name"="x         ") -> ("Signals Out"=w531:dynamicdata)  [unwired: 2 in, 1 out]
                    n405 = xnode "Set Dynamic Data Attributes"("Signals In"=w533, "Signal Name"="y         ") -> ("Signals Out"=w532:dynamicdata)  [unwired: 2 in, 1 out]
                    n406 = xnode "Set Dynamic Data Attributes"("Signals In"=w519, "Signal Name"="max x     ") -> ("Signals Out"=w530:dynamicdata)  [unwired: 2 in, 1 out]
                    n407 = xnode "Set Dynamic Data Attributes"("Signals In"=w518, "Signal Name"="min x     ") -> ("Signals Out"=w529:dynamicdata)  [unwired: 2 in, 1 out]
                    n408 = xnode "Set Dynamic Data Attributes"("Signals In"=w517, "Signal Name"="max y     ") -> ("Signals Out"=w528:dynamicdata)  [unwired: 2 in, 1 out]
                    n409 = xnode "Set Dynamic Data Attributes"("Signals In"=w516, "Signal Name"="min y     ") -> ("Signals Out"=w527:dynamicdata)  [unwired: 2 in, 1 out]
                    n410 = xnode "Set Dynamic Data Attributes"("Signals In"=w520, "Signal Name"="deviation x") -> ("Signals Out"=w524:dynamicdata)  [unwired: 2 in, 1 out]
                    n411 = xnode "Set Dynamic Data Attributes"("Signals In"=w521, "Signal Name"="deviation y") -> ("Signals Out"=w523:dynamicdata)  [unwired: 2 in, 1 out]
                    n412 = xnode "Set Dynamic Data Attributes"("Signals In"=w522, "Signal Name"="trigger count") -> ("Signals Out"=w506:dynamicdata)  [unwired: 2 in, 1 out]
                    n413 = Merge Signals(w531, w532, w530, w529, w528, w527, w524, w523, w506) -> (w535:dynamicdata)
                    n414 = call "Write To Measurement File2"("Signals"=w535, "Filename"="Filename errors") -> ()  [unwired: 15 in, 3 out]
                  }
                }
              }
              frame #6 {
                n415 = local read "data x queue"() -> (w691:i32[])
                n416 = local read "data y queue"() -> (w690:i32[])
                n417 = local read "max x now"() -> (w689:i16)
                n418 = local read "max y now"() -> (w687:i16)
                n419 = local read "min y now"() -> (w686:i16)
                n420 = local read "min x now"() -> (w688:i16)
                n421 = local read "trigger count queue"() -> (w683:i16)
                n422 = call "Convert to Dynamic Data5"("Array"=w691) -> ("Dynamic Data Type"=w673:dynamicdata)  [unwired: 3 in]
                n423 = call "Convert to Dynamic Data6"("Array"=w690) -> ("Dynamic Data Type"=w674:dynamicdata)  [unwired: 3 in]
                n424 = local read "deviation y"() -> (w684:dbl)
                n425 = local read "deviation x"() -> (w685:dbl)
                n426 = xnode "Set Dynamic Data Attributes"("Signals In"=w673, "Signal Name"="x         ") -> ("Signals Out"=w676:dynamicdata)  [unwired: 2 in, 1 out]
                n427 = xnode "Set Dynamic Data Attributes"("Signals In"=w674, "Signal Name"="y         ") -> ("Signals Out"=w675:dynamicdata)  [unwired: 2 in, 1 out]
                n428 = xnode "Set Dynamic Data Attributes"("Signals In"=w689, "Signal Name"="max x     ") -> ("Signals Out"=w677:dynamicdata)  [unwired: 2 in, 1 out]
                n429 = xnode "Set Dynamic Data Attributes"("Signals In"=w688, "Signal Name"="min x     ") -> ("Signals Out"=w678:dynamicdata)  [unwired: 2 in, 1 out]
                n430 = xnode "Set Dynamic Data Attributes"("Signals In"=w687, "Signal Name"="max y     ") -> ("Signals Out"=w679:dynamicdata)  [unwired: 2 in, 1 out]
                n431 = xnode "Set Dynamic Data Attributes"("Signals In"=w686, "Signal Name"="min y     ") -> ("Signals Out"=w680:dynamicdata)  [unwired: 2 in, 1 out]
                n432 = xnode "Set Dynamic Data Attributes"("Signals In"=w685, "Signal Name"="deviation x") -> ("Signals Out"=w681:dynamicdata)  [unwired: 2 in, 1 out]
                n433 = xnode "Set Dynamic Data Attributes"("Signals In"=w684, "Signal Name"="deviation y") -> ("Signals Out"=w682:dynamicdata)  [unwired: 2 in, 1 out]
                n434 = xnode "Set Dynamic Data Attributes"("Signals In"=w683, "Signal Name"="trigger count") -> ("Signals Out"=w692:dynamicdata)  [unwired: 2 in, 1 out]
                n435 = Merge Signals(w676, w675, w677, w678, w679, w680, w681, w682, w692) -> (w672:dynamicdata)
                n436 = call "Write To Measurement File3"("Signals"=w672, "Filename"="Filename history") -> ()  [unwired: 15 in, 3 out]
              }
            }
          }
        }
      }
    }
    n437 = local read "stop"() -> (w226:bool)
    "Numeric" <- w223
  }
  n438 = xnode "Close FPGA VI Reference"("FPGA VI Reference In"=w10, "error in"=w9) -> ()  [unwired: 1 out]
